vi "MAIN - PECT - Autonics - Pulses - encoder - Yokohama.vi"() -> ()   [LabVIEW 2018]
uses:
  Control 1.ctl
  <vilib>/DAQmx/read.llb/DAQmx Read (Counter U32 1Chan 1Samp).vi
  <vilib>/DAQmx/write.llb/DAQmx Write (Analog 1D Wfm NChan NSamp).vi
  <vilib>/DAQmx/read.llb/DAQmx Read (Analog 1D Wfm NChan NSamp).vi
  <vilib>/DAQmx/create/channels.llb/DAQmx Create Channel (AI-Voltage-Basic).vi
  <vilib>/DAQmx/create/channels.llb/DAQmx Create Channel (CI-Count Edges).vi
  <vilib>/DAQmx/miscellaneous.llb/DAQmx Fill In Error Info.vi
  <vilib>/DAQmx/configure/timing.llb/DAQmx Timing (Sample Clock).vi
  <vilib>/DAQmx/configure/trigger.llb/DAQmx Start Trigger (Digital Edge).vi
  <vilib>/DAQmx/create/channels.llb/DAQmx Create Channel (AO-Voltage-Basic).vi
  Global_data.vi
  <vilib>/measure/maspectr.llb/FFT Power Spectrum and PSD for 1 Chan.vi
  <resource>/objmgr/daqmx.rc
  <vilib>/Platform/NI_3dgraph.lvlib
  <vilib>/Instr/_visa.llb/VISA Configure Serial Port (Instr).vi
  <vilib>/measure/NI_MAPro.lvlib
panel:
  out "Array":dbl[][](array[numeric])
  in  "Filter 2":bool
  in  "low cutoff freq: fl 2":dbl=40.0 format="%0.2f"
  in  "Backdata":bool
  out "Numeric 2":i32
  out "Init pulses":i32
  in  "Motor counter":tag="Dev1/ctr0"
  in  "Motor Counter Terminal":tag="PFI8"
  out "dy":dbl[][](array[numeric])
  in  "2D Array In":dbl[][](array[numeric])
  out "Output":dbl[][](array[numeric])
  out "Current  Position (mm)":dbl=12.5
  out "Acquire":bool=TRUE
  out "Numeric":dbl=22.0
  out "Enum":T1(ring)
  in  "Direction (+)":string="+"
  in  "Tab Control 3":enum32{"Control", "Data Processing"}(tab)
  in  "Encoder":bool
  in  "Home":bool
  in  "Exit":bool
  in  "Scan":bool
  in  "Move Dis(mm)":dbl=150.0
  in  "Right":bool
  in  "Forward":bool
  in  "Left":bool
  in  "Backward":bool
  in  "Stop":bool
  in  "Pulser Trigger":tag="/Dev1/PFI0"
  in  "Edge":i32(ring)=10280 items=["Rising"=10280, "Falling"=10171]
  in  "2 Plots":bool
  in  "Offset":bool
  in  "Open csv":bool
  in  "Save Scan mode":bool caption="Save Process"
  in  "Gate 1":dbl
  in  "Gate 2":dbl=20.0
  in  "Open tdms":bool
  in  "Tab Control 4":enum32{"Basic", "Gaussian", "Chirp"}(tab)
  in  "Pulse Basic":T3={"Basic amp"=1.0, "Duty cycle %"=50.0, "Basic freq (Hz)"=200, "Basic Type"=2} {"Basic Type" items=["Sine Wave", "Triangle Wave", "Square Wave", "Sawtooth Wave"]; "Duty cycle %" format="%#.2f"; "Basic amp" format="%0.2p"}
  in  "Pulse Gaussian":T4={"Gauss amp"=2.8, "Gauss Nor. Band"=0.5, "Gauss atten (dB)"=6.0, "Gauss freq (Hz)"=1000.0}
  in  "Pulse chirp":T5={"Chirp amp"=2.1, "Chirp f2"=1500.0, "Chirp f1"=500.0} {"Chirp f1" format="%0.2f"; "Chirp f2" format="%0.2f"; "Chirp amp" format="%0.2f"}
  out "Motor Pulses":i32
  in  "Start idx":i32
  in  "End idx":i32=2000
  in  "Cursor":bool=TRUE
  in  "Repair Line Col":bool
  in  "Repair Line Row":bool
  in  "Line Col":dbl=167.0
  in  "Line Row":dbl
  in  "Y-max":dbl=55.0
  in  "Y-min":dbl
  in  "X-max":dbl=319.0
  in  "X-min":dbl
  in  "Inverse":bool caption="Scan"
  in  "ViewMode":i32(ring) items=["cwViewXYPlane", "cwViewXZPlane", "cwViewYZPlane", "cwViewUserDefined"]
  in  "Plot style":i32(ring)=5 items=["cwLine"=1, "cwPoint"=2, "cwLinePoint"=3, "cwHiddenLine"=4, "cwSurface"=5, "cwSurfaceLine"=6, "cwSurfaceNormal"=7, "cwContourLine"=8, "cwSurfaceContour"=9]
  in  "ColorMapAutoScale":bool=TRUE
  in  "Max":dbl=0.6
  in  "Min":dbl=-0.8
  in  "low cutoff freq: fl":dbl=40.0 format="%0.2f"
  in  "Filter":bool caption="Scan"
  in  "Backindex":i32
  in  "Backdata":bool caption="Scan"
  in  "Odd":bool caption="Scan"
  in  "DiffX":bool caption="Scan"
  in  "DiffY":bool caption="Scan"
  in  "Abs":bool caption="Scan"
  in  "Trim data":bool caption="Scan"
  in  "Return":bool caption="Scan"
  out "No.data":i32
  in  "Tab Control 2":T6(tab)
  out "Hall sensors signal 2":waveform(dbl)(graph)={"t0"=timestamp(3839287492.784824 s since 1904-01-01), "dt"=0.002, "Y"=[], "attributes"=variant("NI_ChannelName"=variant(string "Acquisition Task2"), "NI_UnitDescription"=variant(string "Volts"))}
  out "Hall sensors signal":waveform(dbl)[](graph)=[{"t0"=timestamp(3839287492.7848015 s since 1904-01-01), "dt"=0.002, "Y"=[], "attributes"=variant("NI_ChannelName"=variant(string "Acquisition Task0"), "NI_UnitDescription"=variant(string "Volts"))}, {"t0"=timestamp(3839287492.7848015 s since 1904-01-01), "dt"=0.002, "Y"=[], "attributes"=variant("NI_ChannelName"=variant(string "Acquisition Task0"), "NI_UnitDescription"=variant(string "Volts"))}]
  out "Feature Extraction":dbl(graph)=nan
  out "Power spectral density":cluster{"f0":dbl, "df":dbl, "magnitude":dbl[]}[](graph)=[{"f0"=0.0, "df"=inf, "magnitude"=[]}, {"f0"=0.0, "df"=inf, "magnitude"=[]}]
  in  "Add LF":bool
  in  "Save LF":bool caption="Save Process"
  out "Save Status":bool
  in  "3D Surface (":refnum<k7>(container)
  out "Record path":path=path "H:/Pulsed Eddy Current/PECT_default.tdms" caption="selected path"
  out "Feature extraction scan":dbl[](graph)
  in  "View Mode":bool caption="Scan"
  out "Hall sensors signal lf":dbl[][](graph)=[[-0.70660846198, -0.716567731313, -0.71772803455, -0.717921418426, -0.720596562008, -0.722079171705, -0.724657623384, -0.723561781416, -0.729298836376, -0.728847607304, -0.733553281611, -0.731232675116, -0.734068971955, -0.734230125187, -0.734649123582, -0.735197044564, -0.737292036575, -0.735906118769, -0.738162264033, -0.736454039766, -0.735454889741, -0.737968880154, -0.735422659102, -0.737292036581, -0.734552431644, -0.735809426849, -0.731909518652, -0.731264905752, -0.726591462081, -0.727171613726, -0.72340062815, -0.721080021693, -0.715278505501, -0.71253890069, -0.707188613582, -0.701870557272, -0.697068191179, -0.692362517146, -0.687946918849, -0.677826496722, -0.674571201711, -0.663773936246, -0.660776486438, -0.651622983945, -0.644113244288, -0.636120045089, -0.629867300614, -0.618425422989, -0.610399993434, -0.59950603696, -0.59218968167, -0.58322956384, -0.571207535404, -0.564471331877, -0.553126147145, -0.546615558225, -0.534915836753, -0.528792015616, -0.520315358066, -0.514803919133, -0.504103347861, -0.497753912499, -0.490534250062, -0.48415258421, -0.4781254554, -0.472839631231, -0.469197569495, -0.467811652195, -0.46571666097, -0.462429136198, -0.467457115235, -0.467231500771, -0.474354471106, -0.474741238726, -0.482927820085, -0.490469788806, -0.499204291135, -0.509066865834, -0.523216115386, -0.534432377128, -0.554350911396, -0.569177005115, -0.58816085171, -0.612366062487, -0.634250667901, -0.66187232831, -0.688269225307, -0.719081721676, -0.746928999864, -0.781093486223, -0.813130751347, -0.851227380515, -0.888357092222, -0.928000797226, -0.965807357181, -1.008351826422, -1.048994689492, -1.09189370194, -1.13485717869, -1.180109036257, -1.2251352826, -1.266293851833, -1.314639865003, -1.35380013893, -1.401147008934, -1.441370901989, -1.48307740981, -1.522592234217, -1.561881446939, -1.594208832793, -1.628276678402, -1.656575231322, -1.685228323683, -1.708627813295, -1.726709237842, -1.745338585167, -1.754749951221, -1.765386084343, -1.766481928394, -1.766578620469, -1.759068865834, -1.749141808352, -1.726870391409, -1.702697363978, -1.672142659225, -1.635496354594, -1.591855992024, -1.542736415895, -1.486816169566, -1.426544787201, -1.357119898907, -1.281152192711, -1.205055574576, -1.115615471107, -1.027496838527, -0.924487655795, -0.823476790057, -0.71266782326, -0.598377964549, -0.477738687781, -0.356454816131, -0.226146385508, -0.096933813379, 0.039691785785, 0.177477671952, 0.315553620416, 0.456562543074, 0.59605661768, 0.738386978448, 0.878138885599, 1.019921318004, 1.154935322631, 1.292076548544, 1.418613908244, 1.546504957955, 1.665822671713, 1.781143796386, 1.887472587349, 1.990352709737, 2.080759590593, 2.164752584475, 2.235692182322, 2.298122899903, 2.352689348501, 2.387788500997, 2.419503438832, 2.429204857999, 2.432524612792, 2.418181983039, 2.390753718718, 2.346694452024, 2.29477091497, 2.222380935278, 2.137904477937, 2.035346650361, 1.920347813654, 1.791425361517, 1.644195932762, 1.485299034053, 1.310738069287, 1.125154243505, 0.921650202866, 0.71092650171, 0.483765177519, 0.253445229601, 0.008105779367, -0.246129373952, -0.508261099919, -0.779449723152, -1.058244889529, -1.341584711586, -1.635528585329, -1.928441259944, -2.223868134907, -2.526772774422, -2.823650514512, -3.124106146674, -3.41405481644, -3.706227714753, -3.987442417835, -4.263822791101, -4.527407776882, -4.786577416573, -5.02840704592, -5.262275871216, -5.475098028081, -5.677574208879, -5.860454027961, -6.026509320014, -6.174450790588, -6.300217254762, -6.406645020668, -6.487352250666, -6.552781862445, -6.587011551361, -6.605834660103, -6.593973522799, -6.560743004097, -6.502017506172, -6.420568948967, -6.309918874295, -6.178350774499, -6.019772990024, -5.841921080871, -5.636479455639, -5.407702708707, -5.163100759281, -4.889329996495, -4.60340849308, -4.29102572782, -3.966589007543, -3.624329025262, -3.267791211866, -2.894429352616, -2.512784620922, -2.118957082525, -1.720230866355, -1.310095339563, -0.893610688781, -0.473226398891, -0.047749885035, 0.377081857903, 0.806651402224, 1.226326113266, 1.646645459066, 2.057327931374, 2.465367624173, 2.856937640696, 3.240772514315, 3.608041067282, 3.955230157274, 4.293975068757, 4.609804197942, 4.90271751193, 5.177098363499, 5.426887322034, 5.649860408204, 5.851142279943, 6.021772700426, 6.172194436626, 6.288354759714, 6.38169561436, 6.443353457295, 6.479452149573, 6.483029788153, 6.46127387881, 6.407834927929, 6.330674003129, 6.221217696105, 6.086943623705, 5.925176659162, 5.736206928573, 5.524965806055, 5.286167477957, 5.029771319924, 4.744593282131, 4.446168641795, 4.123506733751, 3.788113950506, 3.432351621052, 3.06650133258, 2.685180548865, 2.296898136162, 1.899107838935, 1.494871524426, 1.086445286821, 0.675762909712, 0.265467248353, -0.150952337452, -0.55870204758, -0.972221258056, -1.373654237756, -1.777923829368, -2.168979184481, -2.552460698049, -2.920729689806, -3.280071163481, -3.622008401497, -3.950860315772, -4.258117910152, -4.550936409787, -4.823256343074, -5.072595856712, -5.304498634402, -5.509682053404, -5.698202166799, -5.859132548236, -6.000240858013, -6.111889905191, -6.206424214181, -6.27008099717, -6.315365963394, -6.333898960157, -6.329676659853, -6.305148642671, -6.25857442753, -6.185216035338, -6.09506518857, -5.986381425725, -5.856360663809, -5.709708700472, -5.54117189352, -5.365641079165, -5.166356100054, -4.957401996174, -4.734878834588, -4.502332058483, -4.25769890765, -4.007715673153, -3.745098175872, -3.482835479658, -3.212193012196, -2.937618633024, -2.664784953904, -2.386601188071, -2.116185239442, -1.843835631437, -1.575257184583, -1.307226809354, -1.048865766862, -0.789924683906, -0.543553647601, -0.298858680926, -0.065186650983, 0.160975596988, 0.377855392589, 0.583937909112, 0.777321550784, 0.961906228802, 1.129988834268, 1.286113886493, 1.434406905534, 1.559977352138, 1.681841284773, 1.782239637185, 1.87196966226, 1.947711605492, 2.009916693762, 2.057166778279, 2.095037754511, 2.114505048262, 2.126913836672, 2.123561852274, 2.106834160961, 2.083724807448, 2.04517698859, 1.999828510872, 1.941362174369, 1.876127411384, 1.800417702224, 1.720518017024, 1.626759173182, 1.53477301667, 1.432666452766, 1.3256930704, 1.216753623473, 1.100658983649, 0.982533816097, 0.864892106737, 0.741448886061, 0.618489120633, 0.497011957912, 0.371215886709, 0.252865078568, 0.127455756566, 0.00929831228, -0.108053378055, -0.221569636608, -0.333216531681, -0.440351151746, -0.547066787125, -0.643984321714, -0.742481170629, -0.834016212751, -0.919943133402, -1.004129610016, -1.078743591058, -1.154131117554, -1.220526296559, -1.28176457554, -1.335299729295, -1.389318348703, -1.430928160202, -1.472151206875, -1.504381894686, -1.533711822363, -1.557723687612, -1.576417489536, -1.58798830868, -1.597464132915, -1.601750815379, -1.601621892616, -1.59852774587, -1.588246154234, -1.580027327232, -1.560882295453, -1.54560494743, -1.52268892626, -1.50177120885, -1.474117278751, -1.447236886611, -1.415296278632, -1.385869665753, -1.349996918726, -1.315800169399, -1.280926577982, -1.245472836775, -1.210728172549, -1.170472066246, -1.137048863988, -1.097276222791, -1.065400096546, -1.027077839927, -0.994814949512, -0.958942227201, -0.927646259992, -0.892128078709, -0.861283343899, -0.830664225057, -0.801817793355, -0.772777978979, -0.746928999873, -0.722723784605, -0.697132652466, -0.677504190288, -0.654072512801, -0.640019952773, -0.620713798494, -0.607112468066, -0.589804614323, -0.577589201926, -0.565986171871, -0.555930212629, -0.54590648416, -0.539105819592, -0.533239843546, -0.528050710938, -0.523635113662, -0.51996082103, -0.521346738438, -0.518703826188, -0.521314507795, -0.519896359761, -0.525472259972, -0.524408648935, -0.530177933006, -0.532079540602, -0.538815743842, -0.541813193149, -0.548871702871, -0.55319060837, -0.559572274784, -0.565953941223, -0.570885229012, -0.57865281302, -0.584647711969, -0.594349134521, -0.597120969574, -0.607305851908, -0.611399143265, -0.6213584113, -0.626902081599, -0.634282898507, -0.640019952747, -0.647046232714, -0.651300677507, -0.657295577056, -0.662162404096, -0.668737455294, -0.674216664635, -0.675602582331, -0.683531320648, -0.684949468998, -0.693136052559, -0.694167433224, -0.700516870141, -0.703095321724, -0.708961299059, -0.708219994242, -0.711443058732], [-0.711700903907, -0.720274255531, -0.721080021681, -0.724464239466, -0.722433708801, -0.725141083016, -0.72559231207, -0.726204694336, -0.729202144406, -0.727848457275, -0.731039291205, -0.729975679907, -0.73139382833, -0.73123267509, -0.734165663872, -0.732392978358, -0.735648273607, -0.732908668699, -0.73590611877, -0.734810276807, -0.73352105101, -0.733843357422, -0.732844207425, -0.733230975136, -0.731007060611, -0.73062029283, -0.728106302452, -0.729427758908, -0.724174163692, -0.726043541112, -0.72166017329, -0.721208944256, -0.715181813577, -0.712248824884, -0.70754315068, -0.704739084581, -0.697809495981, -0.693361667074, -0.688849376879, -0.681694173927, -0.676311656471, -0.666481310252, -0.663677244331, -0.654942740122, -0.649270147063, -0.638827419012, -0.632703597094, -0.62161625644, -0.613816441327, -0.601891104324, -0.593382215333, -0.583906407255, -0.574301676729, -0.564729176965, -0.553480684115, -0.54616432927, -0.535624910724, -0.527373867557, -0.517382370077, -0.511258549117, -0.498881984754, -0.493789544277, -0.484603813104, -0.479898140329, -0.472710708686, -0.46910087758, -0.464072898546, -0.462042368558, -0.459721762867, -0.45836807625, -0.458948227649, -0.460366375577, -0.465104278851, -0.467167039506, -0.476352770465, -0.481703055936, -0.495368845435, -0.504619038035, -0.520702125685, -0.534819144789, -0.554447603261, -0.570530691961, -0.592511988075, -0.615621357208, -0.640535643041, -0.667319306976, -0.694973199311, -0.727912918571, -0.7584675715, -0.795017126404, -0.828988231267, -0.870404618505, -0.908050021807, -0.951432484146, -0.989754736086, -1.033685125354, -1.077228749861, -1.121674836208, -1.166572155322, -1.211276093955, -1.257140340429, -1.302521130597, -1.347934155322, -1.389930731637, -1.437535450536, -1.478565113577, -1.521947620419, -1.557949302468, -1.598431053803, -1.629565906268, -1.663762677273, -1.691223234113, -1.718941638241, -1.740310595099, -1.759874633465, -1.772831377568, -1.782081590668, -1.788237655914, -1.788173194541, -1.784176586682, -1.7728636083, -1.758134175287, -1.733090917251, -1.706693971085, -1.669886510205, -1.632917898781, -1.584314009521, -1.53206805716, -1.471442131748, -1.407141915873, -1.333398119264, -1.254561886613, -1.168796071461, -1.07871136044, -0.983147451101, -0.877076363675, -0.77200444347, -0.655490661079, -0.541426425506, -0.414760028952, -0.290317564379, -0.158687687189, -0.026832212351, 0.113370977212, 0.253509690839, 0.395968995891, 0.538202675996, 0.682209031094, 0.82640876359, 0.965999515658, 1.107943100394, 1.2432149505, 1.379195876537, 1.506635696159, 1.632560682823, 1.748236342269, 1.865201233481, 1.969338348306, 2.067416114716, 2.15692054372, 2.236530178481, 2.30560040478, 2.364485757723, 2.409930942223, 2.44470779056, 2.468332842109, 2.474327739345, 2.470137757407, 2.448124237269, 2.417408447956, 2.366355134083, 2.304955792292, 2.22576515062, 2.134197956683, 2.022454403625, 1.899978065497, 1.759420364327, 1.606872887466, 1.438564653815, 1.256074962083, 1.059951729476, 0.851161868759, 0.630478906609, 0.399030903911, 0.159009529445, -0.095741280337, -0.355101129604, -0.628997073303, -0.906148413194, -1.193065765257, -1.484979020361, -1.782984050494, -2.083052046727, -2.385956572993, -2.689473733606, -2.994473784422, -3.295767585382, -3.589680826897, -3.885270392832, -4.167097682705, -4.447442674322, -4.711382413403, -4.969939881134, -5.21305896681, -5.445155293591, -5.65475453306, -5.853298698642, -6.032053093797, -6.193563935177, -6.333222102904, -6.451672172544, -6.551138064005, -6.625721405834, -6.678709764359, -6.705397338156, -6.7118436127, -6.689732892102, -6.647219721964, -6.571991743565, -6.476812606234, -6.354849306761, -6.207552308847, -6.03563076211, -5.840825219647, -5.620911798473, -5.380693017663, -5.114625193963, -4.828993469243, -4.526666463854, -4.200843492433, -3.861516208625, -3.502302924475, -3.13216385381, -2.744427224852, -2.350406050506, -1.943944235937, -1.534034129331, -1.111328792601, -0.688108072092, -0.254348183817, 0.180185043615, 0.614653678333, 1.048574325895, 1.479626447166, 1.903394510606, 2.321264488474, 2.731753822843, 3.124806592014, 3.511768013492, 3.874782309212, 4.221391454251, 4.556655670645, 4.868101642753, 5.155503714809, 5.423470852265, 5.66481553335, 5.882245096744, 6.070795930585, 6.233626609533, 6.371091627426, 6.475326584487, 6.555807348401, 6.601285277357, 6.622976737884, 6.609955415071, 6.570891451368, 6.499628742443, 6.407544849292, 6.28052263845, 6.128070288235, 5.948608528303, 5.743491108137, 5.514426315553, 5.258964657354, 4.982101962969, 4.683548195569, 4.366655388863, 4.026975726542, 3.675113132109, 3.302687625615, 2.924912076204, 2.52876527563, 2.127365065353, 1.717166033533, 1.303228338131, 0.883199090654, 0.465587113791, 0.041722314718, -0.374858506392, -0.792632058415, -1.209664560433, -1.619703313065, -2.022973968836, -2.416640254231, -2.801153418931, -3.170164003204, -3.529376856542, -3.867414465728, -4.195654308351, -4.499141189584, -4.786964188961, -5.051871271029, -5.297149939141, -5.518352233991, -5.717154105289, -5.893104251006, -6.046299304766, -6.173645008773, -6.275238003521, -6.35791128069, -6.408675593623, -6.444194505839, -6.448062264612, -6.433687095446, -6.394268196495, -6.335252674733, -6.248389341404, -6.145345955566, -6.020353152397, -5.879180364564, -5.71757311064, -5.538109933487, -5.346721406584, -5.136058870085, -4.916694164197, -4.681472020658, -4.438804768894, -4.185340402521, -3.926783816261, -3.653465746224, -3.381437188134, -3.103252801735, -2.823908360859, -2.542275774546, -2.258999645662, -1.980912873448, -1.705791511432, -1.431605004604, -1.161544171119, -0.901281584442, -0.641986021923, -0.394615883648, -0.147374738228, 0.083364272888, 0.312008253063, 0.526470734451, 0.730973938979, 0.921811355892, 1.10391427476, 1.267806902505, 1.422997270747, 1.563135951752, 1.687868408833, 1.801094545084, 1.89701284902, 1.981811596561, 2.050430579225, 2.106834160953, 2.147799278231, 2.17816052264, 2.190633772981, 2.194823753727, 2.183317421989, 2.162238596067, 2.128299753321, 2.084208266714, 2.0311889008, 1.967017743996, 1.893370789696, 1.81256864297, 1.725739375948, 1.627307093536, 1.528359125728, 1.41655114942, 1.30799846779, 1.188100615371, 1.068557301022, 0.944695085629, 0.822992319382, 0.695069043221, 0.570272131299, 0.442284382926, 0.317616379586, 0.194624359058, 0.068441497018, -0.050553949051, -0.171128708146, -0.285160663856, -0.399676092901, -0.508132177389, -0.615073436322, -0.712184363585, -0.810874605876, -0.899960127607, -0.986692823527, -1.067462858994, -1.142721461342, -1.214112393046, -1.278251431973, -1.337298031367, -1.389382810045, -1.440339520092, -1.481240260618, -1.520884007654, -1.548602401773, -1.57802902429, -1.595723675412, -1.612902636098, -1.621959461795, -1.628502293261, -1.629275830005, -1.627986602099, -1.618188470277, -1.608358107981, -1.59524021497, -1.575482799408, -1.556627844048, -1.531455674043, -1.507895039751, -1.477243655394, -1.44794596169, -1.414168204733, -1.38277552038, -1.345710238439, -1.31270602436, -1.274061444278, -1.238059782054, -1.200704434038, -1.16164086315, -1.124865672142, -1.086188874377, -1.050283915983, -1.013218656049, -0.978731850936, -0.941376519413, -0.91175654708, -0.874530142074, -0.846586166678, -0.814258824097, -0.786379312543, -0.757500652045, -0.731554981564, -0.705641542641, -0.684433778674, -0.659003801079, -0.639955491476, -0.622712098238, -0.603212560587, -0.590352535192, -0.573463680108, -0.562601954829, -0.551933613494, -0.542554497827, -0.532853075905, -0.529694473448, -0.52025089677, -0.519058363199, -0.513837000046, -0.511451932947, -0.512870080968, -0.511838700566, -0.511677547393, -0.514352690234, -0.517285678205, -0.520508741861, -0.526568101624, -0.527825096497, -0.538493437484, -0.540427275726, -0.547389093516, -0.553061685838, -0.559540044149, -0.566147325069, -0.57620328444, -0.578652813016, -0.588676541915, -0.596540818049, -0.602116718805, -0.61207598672, -0.616749429656, -0.626450852631, -0.6339605921, -0.639955491487, -0.645563623199, -0.654459280486, -0.657263346399, -0.666739155394, -0.66922091493, -0.67573150487, -0.681823096537, -0.68501393027, -0.690783215552, -0.69532773638, -0.698035110534, -0.70357878138, -0.706382847481, -0.706995229747, -0.714827276494, -0.711829826488, -0.717115652296], [-0.710927368415, -0.721563481368, -0.721595712031, -0.723303936229, -0.725108852432, -0.725527850816, -0.729427758978, -0.727300536363, -0.732876438089, -0.733166513892, -0.737034191399, -0.735003660722, -0.738549031766, -0.738452339841, -0.737968880135, -0.738903568875, -0.741095252863, -0.738645723707, -0.741030791566, -0.739677104411, -0.739354797941, -0.742094402897, -0.73774326562, -0.742932399702, -0.737743265618, -0.738968030203, -0.735519351038, -0.735035891386, -0.730845907349, -0.72978229604, -0.724464239482, -0.723819626589, -0.716019810351, -0.714408278121, -0.708574531326, -0.703063091172, -0.698679723421, -0.692878207473, -0.688398147883, -0.678213264461, -0.674829046864, -0.664257395879, -0.659519491377, -0.650656064667, -0.642179405778, -0.633799438886, -0.625226088263, -0.614525515429, -0.606081087604, -0.593478907265, -0.587516238926, -0.577041281088, -0.564471331913, -0.558605355655, -0.545197410173, -0.540781812775, -0.528276325465, -0.521250046516, -0.512773389061, -0.505295881372, -0.496013458178, -0.490598711337, -0.480768367493, -0.477255228246, -0.470325641713, -0.466393504254, -0.46226798305, -0.458819305132, -0.460559759439, -0.456659852641, -0.462429136215, -0.463879514767, -0.471389252665, -0.472517324904, -0.483153434512, -0.490502019438, -0.50084805357, -0.513160156676, -0.528147402851, -0.542361113995, -0.561699496934, -0.579780885408, -0.602664639692, -0.627611155718, -0.650108143758, -0.682467709413, -0.707704303918, -0.742610093227, -0.773390361308, -0.810391146154, -0.844877942157, -0.884070415338, -0.922714969748, -0.965130513384, -1.004194071312, -1.050251685316, -1.092699468449, -1.135695176079, -1.183235411066, -1.227133584269, -1.276382052832, -1.317637317973, -1.366466795995, -1.408012144306, -1.454714405619, -1.494777149486, -1.537934042904, -1.57635302815, -1.614095171865, -1.647905173327, -1.679620181747, -1.706984047416, -1.734025607719, -1.755845795159, -1.771058688734, -1.787077350425, -1.793910260671, -1.803063782041, -1.796939947333, -1.794844951197, -1.782500589886, -1.765353853546, -1.740826286392, -1.711657499304, -1.673367425821, -1.633207975063, -1.581703323307, -1.527845836705, -1.464705918282, -1.396151253222, -1.324856989698, -1.238930010223, -1.155291421567, -1.061242341096, -0.964228054985, -0.855095058719, -0.747960380555, -0.628481383047, -0.509260249656, -0.382271551645, -0.252317654314, -0.117787026094, 0.01909642047, 0.16013760098, 0.300663077532, 0.445829750017, 0.592833556893, 0.73248877748, 0.882199941889, 1.021210542207, 1.165829267176, 1.303453952372, 1.438274578348, 1.570484530423, 1.696796287823, 1.813857867449, 1.930307073514, 2.031124439534, 2.130330282341, 2.219673563048, 2.293578381865, 2.362261844503, 2.416119222821, 2.462434636828, 2.491828971774, 2.511876424447, 2.513326802871, 2.507525289189, 2.480902787945, 2.44390202482, 2.389980183652, 2.321103335349, 2.237626019648, 2.138613551575, 2.020552797226, 1.892371640636, 1.746141352558, 1.583860232908, 1.41087856266, 1.216528009233, 1.019792395584, 0.801139968617, 0.572592735082, 0.334891987588, 0.086426181539, -0.174448462454, -0.439416463364, -0.719307336175, -1.001099928024, -1.292304006338, -1.591630377162, -1.893019701465, -2.201209923647, -2.506660775153, -2.815625046101, -3.122430143612, -3.429364475269, -3.72505055753, -4.023057597177, -4.307076750992, -4.584972354295, -4.851974206402, -5.106148417387, -5.347559415797, -5.576948483823, -5.784839614889, -5.981159965478, -6.156111198496, -6.30959656147, -6.45041515099, -6.55987275788, -6.655793263995, -6.722995668099, -6.76869976497, -6.787490663209, -6.783590665282, -6.752519610718, -6.698564287283, -6.615794148269, -6.511880294189, -6.378281466584, -6.220025813415, -6.041238998862, -5.833121960323, -5.605054062077, -5.350234599383, -5.079590001991, -4.780034515432, -4.468360588381, -4.130322168267, -3.780036472621, -3.411089577322, -3.030185528628, -2.634907020607, -2.231700205315, -1.816117219547, -1.398761938448, -0.967870119262, -0.533948917579, -0.10031802868, 0.342014952778, 0.778997542299, 1.221878289721, 1.653542809478, 2.083595884971, 2.502368388148, 2.912342123176, 3.308199069955, 3.69280778213, 4.05759490835, 4.402173670004, 4.736986818805, 5.045499953056, 5.330420413114, 5.590007684748, 5.831030201483, 6.037340233968, 6.223796171648, 6.375088266782, 6.505817090897, 6.600028268508, 6.67061415748, 6.707615353626, 6.71873505223, 6.697236968676, 6.649148309384, 6.567990662195, 6.460919338063, 6.323744347412, 6.159398755148, 5.970042083259, 5.748390202495, 5.509785072288, 5.239207160015, 4.951933935452, 4.638650733591, 4.311863128522, 3.962482067337, 3.598823090781, 3.219435814265, 2.828187905105, 2.423532267353, 2.013268677874, 1.593787260336, 1.170857241583, 0.745058713974, 0.317455226524, -0.10628069381, -0.536559599228, -0.956170390698, -1.37877891595, -1.790010344895, -2.197890157421, -2.592974779821, -2.979196378686, -3.349786489195, -3.70845164637, -4.045715944667, -4.3717965508, -4.673607650656, -4.956273909006, -5.2199564235, -5.459272535097, -5.679089074392, -5.868286213282, -6.041658005013, -6.18408794079, -6.30775937747, -6.402938419599, -6.474846495158, -6.520550523301, -6.54420832557, -6.539824863307, -6.514362106984, -6.463887844289, -6.3946872037, -6.301667662811, -6.18431355981, -6.054260422905, -5.897584390787, -5.732012684015, -5.54088181332, -5.340758648073, -5.123682130552, -4.894293578911, -4.649466615545, -4.398161494277, -4.134189881976, -3.865738458211, -3.588165975379, -3.308531000887, -3.0243839815, -2.736756297111, -2.452932090653, -2.16456357347, -1.884962022521, -1.602911120461, -1.331432047928, -1.056794509731, -0.793631208497, -0.533046459727, -0.280068224611, -0.036372475961, 0.196300351006, 0.424912084094, 0.636344877161, 0.841073689194, 1.031073107354, 1.206472060374, 1.373845595888, 1.519656861632, 1.659795547723, 1.778468655645, 1.889341962949, 1.981070292399, 2.061356758571, 2.12433538713, 2.176226685399, 2.211293601344, 2.236240102863, 2.244781217885, 2.243040764236, 2.228472522925, 2.201495492363, 2.160498142613, 2.110605143374, 2.055104018764, 1.981038061762, 1.907165492431, 1.816758622552, 1.72515922494, 1.623342728618, 1.517207335446, 1.405012592267, 1.290142712201, 1.168246562564, 1.047156179274, 0.919039523837, 0.792727780462, 0.665803652141, 0.534979615125, 0.407733168748, 0.276586809842, 0.152950173688, 0.024575625662, -0.097675117694, -0.219539107163, -0.33276530288, -0.44750635248, -0.555833520716, -0.659648413935, -0.759434490888, -0.85722228175, -0.945888811272, -1.032557052242, -1.113939476566, -1.187393167446, -1.260202254478, -1.321988459376, -1.383935824916, -1.431895080745, -1.481530336808, -1.52059393143, -1.554532849089, -1.584926392742, -1.610227488406, -1.62624614447, -1.64239372398, -1.647872942625, -1.65280423958, -1.652836470222, -1.645584563108, -1.639911960213, -1.625472607776, -1.610549795346, -1.5874726176, -1.567940817251, -1.540705882338, -1.514212254869, -1.483045179111, -1.452554949714, -1.416521044576, -1.38277552039, -1.345001163501, -1.307291270799, -1.268163230894, -1.23274172125, -1.193581455997, -1.150585744158, -1.117291465704, -1.074875911501, -1.041484945369, -1.003001536946, -0.967515582024, -0.932223013107, -0.898219672272, -0.863507258885, -0.833178215835, -0.799142649494, -0.772745748364, -0.743351398115, -0.716471039411, -0.693587281637, -0.668092842444, -0.650688295345, -0.627256618724, -0.612881752772, -0.595863974652, -0.583519639569, -0.56724316682, -0.556800439871, -0.545551947147, -0.535721602628, -0.528276325388, -0.523796266856, -0.516060913979, -0.514094845139, -0.511065165314, -0.508841251385, -0.512032084435, -0.509002404553, -0.516350989715, -0.514513843417, -0.520831048233, -0.522764886451, -0.526729254832, -0.53195061806, -0.538590129407, -0.541652039967, -0.550966694366, -0.553802990491, -0.563053183779, -0.569853848527, -0.575590902357, -0.584905557093, -0.590932686735, -0.601020877055, -0.60350263635, -0.614944513774, -0.618908882582, -0.629125995866, -0.634927511342, -0.643146325024, -0.647884229412, -0.655651814247, -0.659551722015, -0.665675544213, -0.668963069777, -0.677633112898, -0.681629712678, -0.682854477157, -0.691717904228, -0.692169133285, -0.701097021755, -0.701580481458, -0.70715638295, -0.710379447476, -0.713634742606, -0.714279355512, -0.718340416815], [-0.711765365224, -0.724560931444, -0.722369247503, -0.726784845983, -0.72494769918, -0.728621992799, -0.727880687945, -0.730072371842, -0.730169063782, -0.730845907354, -0.730104602467, -0.732618592899, -0.730749215401, -0.73229628649, -0.731135983188, -0.734230125256, -0.735744965582, -0.730781446088, -0.737066422059, -0.732747515477, -0.736228425243, -0.735197044577, -0.734326817112, -0.734584662293, -0.73342435903, -0.730555831519, -0.730684754112, -0.725270005612, -0.726108002436, -0.721885787838, -0.717824726532, -0.717147883005, -0.710476139452, -0.711249674934, -0.703578781432, -0.702676323345, -0.696004579975, -0.692813746133, -0.684240394829, -0.67934133696, -0.672121672803, -0.663354937875, -0.655812967451, -0.650043682499, -0.638440651315, -0.632123445558, -0.622744328924, -0.611689219083, -0.607595927736, -0.593865674939, -0.589933536879, -0.575333057211, -0.567501011901, -0.558411971797, -0.547131248426, -0.538364514917, -0.530081241095, -0.517382370075, -0.51100070404, -0.498624139668, -0.492371396341, -0.485183964551, -0.476449462421, -0.473194168256, -0.465555507761, -0.464234051759, -0.457014389609, -0.457755694206, -0.454371477587, -0.456530930071, -0.456982158954, -0.458819305118, -0.462396905535, -0.46897195505, -0.47374208902, -0.483926969825, -0.492210243146, -0.508003254901, -0.522893809026, -0.535270373741, -0.558895431386, -0.574559521866, -0.601278722161, -0.624001323916, -0.650913909799, -0.679824796629, -0.710411678102, -0.740547331832, -0.775582045369, -0.808135000648, -0.848326621873, -0.884908412339, -0.925744651385, -0.968127964584, -1.008577441074, -1.056762279125, -1.097276222847, -1.147588292081, -1.191615385176, -1.241476233341, -1.284697567014, -1.33227004555, -1.378778915937, -1.420968878904, -1.465318301289, -1.510505725619, -1.547055328546, -1.589825458321, -1.625085839421, -1.659056995213, -1.6933182298, -1.717781332923, -1.748690578516, -1.765740622068, -1.785755891413, -1.798164714248, -1.806254622338, -1.809703308258, -1.809252078319, -1.799163866215, -1.788269886665, -1.76541831494, -1.743694819196, -1.711302961563, -1.672851734771, -1.630113828191, -1.577964562881, -1.525267381534, -1.456487093395, -1.391864572571, -1.311513489345, -1.230872342166, -1.140529775998, -1.045288163425, -0.943826049219, -0.836916971325, -0.721821326526, -0.606467855284, -0.479189066374, -0.355326744083, -0.223052245422, -0.083783719617, 0.049554354938, 0.196719348996, 0.334666373306, 0.48295941228, 0.627545921343, 0.774259643201, 0.919458521707, 1.065463162938, 1.206891058243, 1.34793218853, 1.481882589672, 1.615349537597, 1.739276232442, 1.860205488455, 1.972754793568, 2.073636624006, 2.174131695086, 2.255288400978, 2.334833581771, 2.396265156012, 2.453506752411, 2.495084265497, 2.524027372682, 2.541045146617, 2.543430213434, 2.529861117134, 2.506655062122, 2.462015638659, 2.408770639614, 2.335897192413, 2.24555475284, 2.146123286002, 2.021197409573, 1.891179107926, 1.737793624341, 1.575093507418, 1.394763259411, 1.202088698055, 0.994652523619, 0.776225710175, 0.544100877349, 0.304208444897, 0.047813901563, -0.211159144441, -0.483798047303, -0.7653326994, -1.052572293041, -1.351124992534, -1.647808481302, -1.959221597519, -2.263576411537, -2.577342854314, -2.887370806551, -3.196786672335, -3.502560771377, -3.804693114694, -4.097801143999, -4.386429416404, -4.661940020556, -4.932841925659, -5.185952608819, -5.425397603927, -5.655914855497, -5.862258976218, -6.060545516593, -6.229662966251, -6.387080614154, -6.520099284844, -6.631684206844, -6.718579969795, -6.784170830334, -6.823106351241, -6.840704694108, -6.828811308327, -6.796128675609, -6.733793179361, -6.64683294574, -6.537890983214, -6.395138442166, -6.238010868241, -6.046911698304, -5.838214491566, -5.598736752886, -5.34024295002, -5.058736491301, -4.756151316888, -4.432584187887, -4.093063195321, -3.731174427893, -3.358005356716, -2.96743213227, -2.568350468634, -2.160405808323, -1.73857013707, -1.318604238285, -0.881105195248, -0.447989812003, -0.002143557587, 0.439770395346, 0.884520545481, 1.326466604942, 1.764770645786, 2.195178290564, 2.620235815048, 3.02843692896, 3.430288857773, 3.814124125672, 4.179072505695, 4.52316791251, 4.853211018603, 5.164689498048, 5.44345397781, 5.704814050875, 5.9364897071, 6.144959296661, 6.322745187771, 6.475552201279, 6.596772938093, 6.691693235321, 6.755704025392, 6.790030060846, 6.791222608696, 6.766114644038, 6.710580606664, 6.62197757689, 6.508234414488, 6.359295095206, 6.193789165152, 5.98938063049, 5.765923803883, 5.515522164724, 5.241753395342, 4.94510100651, 4.628981503492, 4.290397456829, 3.93847018769, 3.564207334467, 3.179985482758, 2.78126008812, 2.368385663559, 1.953803191747, 1.525587293446, 1.098338380085, 0.665416884865, 0.236459696272, -0.197138822371, -0.624291399669, -1.052507831657, -1.472989204735, -1.890312321264, -2.296774081073, -2.696242198286, -3.081722610934, -3.457050786674, -3.813749999477, -4.153560682818, -4.479544743602, -4.778809735956, -5.065569480639, -5.322515831455, -5.562960158558, -5.776523965273, -5.966945991103, -6.133227000213, -6.275431391187, -6.390561595666, -6.484773744206, -6.547657079024, -6.589880141444, -6.607413996422, -6.599259464388, -6.570734721027, -6.512073682302, -6.438199480229, -6.338024566655, -6.220122507215, -6.078304936196, -5.921564420508, -5.743229139087, -5.550132156053, -5.341113190445, -5.117300374375, -4.880176376789, -4.633899033522, -4.373504792794, -4.106825808411, -3.833475315589, -3.551261620261, -3.269950678431, -2.976327836394, -2.691053042014, -2.398881106403, -2.110996091378, -1.823433590916, -1.540995958539, -1.262200556184, -0.990302657263, -0.720725484573, -0.461558909037, -0.206614626238, 0.037919101747, 0.272267907717, 0.499590406638, 0.709766199878, 0.914688392123, 1.100852367279, 1.279925610207, 1.440724104466, 1.590016279132, 1.724740227003, 1.845605020756, 1.949516519928, 2.042534077976, 2.117470265228, 2.181157970384, 2.227731218564, 2.261766756197, 2.283038967805, 2.28664879767, 2.282748892171, 2.259220536969, 2.232630273161, 2.185960332916, 2.134133495452, 2.069672257958, 1.998023596367, 1.916286756241, 1.827588108294, 1.729381434927, 1.628402934234, 1.516723876331, 1.403529984368, 1.285275890746, 1.159995527641, 1.038131609861, 0.904245675988, 0.777353781392, 0.643338918953, 0.515641249901, 0.383495749512, 0.254637762314, 0.12616653192, 0.001015043127, -0.123491846328, -0.242132776215, -0.360709259352, -0.471582636471, -0.580715573951, -0.687463459203, -0.785315701171, -0.884682797774, -0.971737798179, -1.062015877006, -1.138015783997, -1.214273546373, -1.282054651605, -1.345678007751, -1.402500697588, -1.453940869169, -1.497774603487, -1.539384423977, -1.570196965704, -1.599140129151, -1.621701616217, -1.638977270006, -1.65506038846, -1.657896689984, -1.66540644294, -1.659475994245, -1.6561884629, -1.644843256998, -1.631628670883, -1.614481940201, -1.594917908013, -1.569326736977, -1.543928951467, -1.513599871748, -1.483303024612, -1.44929965047, -1.4141037433800001, -1.380390449999, -1.340682252615, -1.307678038826, -1.264521164743, -1.230131036731, -1.189617083625, -1.151584894783, -1.112360173922, -1.07342553161, -1.034780967818, -0.998328091321, -0.959328995068, -0.926228111175, -0.88954962641, -0.857383435016, -0.825056091908, -0.790665988836, -0.767621075384, -0.735583812304, -0.713473589391, -0.685658543145, -0.665159853888, -0.642662865403, -0.622808790165, -0.604050557231, -0.587870775927, -0.571852148146, -0.55921773777, -0.545165179484, -0.536269523486, -0.526535870989, -0.517736907139, -0.515287378725, -0.507165258283, -0.507906562927, -0.501395974404, -0.503748810838, -0.50236289347, -0.504393423551, -0.505682649001, -0.508293330553, -0.510388321916, -0.515867530145, -0.518059213454, -0.524569802165, -0.52875978496, -0.535786063969, -0.544327182925, -0.5475180161, -0.558959892661, -0.561989572689, -0.574462829917, -0.58013542245, -0.588805464462, -0.597636659824, -0.605597627963, -0.612591676972, -0.619392342204, -0.625580625296, -0.63495974198, -0.639891030191, -0.646466081183, -0.654330357939, -0.658165804432, -0.668737455312, -0.669672143973, -0.680662793387, -0.683982549693, -0.691427828421, -0.694360817091, -0.698679723403, -0.703030860409, -0.706511770053, -0.708606761965, -0.712861207147, -0.712990129697, -0.717695803943, -0.718082571675], [-0.71427935551, -0.722143632976, -0.72404524108, -0.724464239483, -0.726011310473, -0.728170763755, -0.726236924985, -0.730974829944, -0.729911218611, -0.734423509066, -0.732006210595, -0.73532596716, -0.734326817122, -0.73645403979, -0.734487970348, -0.737324267224, -0.735809426843, -0.737130883336, -0.735616042946, -0.735841657505, -0.735809426825, -0.734004510669, -0.735325967138, -0.73245743967, -0.733005360631, -0.72833191696, -0.728944299233, -0.724367547531, -0.724883237855, -0.721015560384, -0.718179263577, -0.713151282924, -0.711636442602, -0.704996929745, -0.70048463953, -0.69590788798, -0.690009680114, -0.685787465724, -0.676247195206, -0.67276628568, -0.662742555697, -0.659003801098, -0.648496611662, -0.643371939515, -0.635346509704, -0.629125995852, -0.617587426319, -0.609626458033, -0.598313503252, -0.590062459426, -0.5810056497, -0.569982771092, -0.560764808435, -0.550934463727, -0.54278011233, -0.530435778128, -0.525568951902, -0.515126225547, -0.509163557759, -0.49820514143, -0.491275554701, -0.483862508508, -0.476868460633, -0.470647948067, -0.466232351115, -0.461107680184, -0.458625921328, -0.455628472316, -0.453501250461, -0.455789625498, -0.455499549774, -0.462267983033, -0.463879514753, -0.471679328402, -0.477351920158, -0.487569031621, -0.495787843706, -0.511451932955, -0.524118573203, -0.541361964245, -0.557606205819, -0.579490809668, -0.601020877026, -0.62522608831, -0.651203985583, -0.68021156439, -0.710701753907, -0.739967180224, -0.77648450352, -0.809585379893, -0.849261310757, -0.886810020881, -0.928903255565, -0.969288268192, -1.013669885247, -1.056182127116, -1.102239745154, -1.14662137207, -1.194193838741, -1.239993622437, -1.283891800131, -1.333108043207, -1.377167381948, -1.425126637116, -1.467606680147, -1.512761873853, -1.55398492737, -1.595369137754, -1.630146058852, -1.665793211348, -1.697089221818, -1.725935700923, -1.7511078814, -1.771961148467, -1.789784729985, -1.802322475745, -1.811443766655, -1.812088380825, -1.814022223456, -1.80486870181, -1.794780489812, -1.772154532753, -1.749109577661, -1.716040874956, -1.677847493227, -1.632305515562, -1.582380167971, -1.52243108076, -1.459226701699, -1.386159741905, -1.308967265931, -1.22658566283, -1.13463156401, -1.040292410915, -0.936348537068, -0.829181615174, -0.712764515191, -0.595606129522, -0.467747190914, -0.342724567549, -0.20651793436, -0.070891470967, 0.071600097559, 0.213414807264, 0.359129407496, 0.506584448778, 0.654297325408, 0.800882123762, 0.94737022586, 1.096952464068, 1.236027525487, 1.379518182597, 1.512469436124, 1.645259542865, 1.769379623202, 1.890341111973, 2.001085504894, 2.107930002, 2.202365719158, 2.290387550084, 2.363937837082, 2.429043704874, 2.484931616791, 2.523350529433, 2.553260556559, 2.564992507132, 2.567732111023, 2.551584563608, 2.522383610465, 2.476454960925, 2.420470357663, 2.343825926324, 2.255417323432, 2.149281886744, 2.02712784304, 1.88930973233, 1.737761393734, 1.570162224343, 1.387124605696, 1.192451747079, 0.979407447398, 0.758434415577, 0.519895690267, 0.278069418051, 0.018709653029, -0.244840148886, -0.519219516403, -0.800979796488, -1.094955614997, -1.389286118006, -1.694833072763, -2.000702537671, -2.312986148011, -2.625850171815, -2.93652278559, -3.249355170025, -3.556031789992, -3.859840201111, -4.153141680389, -4.444058420266, -4.719923636027, -4.989923143988, -5.243775212777, -5.485573151627, -5.709837625206, -5.920081784168, -6.110826273553, -6.282651200402, -6.433461476219, -6.566415720895, -6.675067619843, -6.758450185193, -6.824588995507, -6.859173286962, -6.875772460093, -6.859624526589, -6.824137755937, -6.759191506871, -6.670909773554, -6.553490951991, -6.413091283668, -6.242394322554, -6.052036466714, -5.835281451458, -5.593354147693, -5.330863692688, -5.043555652639, -4.739294486152, -4.410602654685, -4.067600751817, -3.704519477413, -3.328385203867, -2.933009627492, -2.530962774319, -2.115669547686, -1.693124845495, -1.263489783148, -0.828827078002, -0.386300380611, 0.058256621803, 0.505617530523, 0.952494892089, 1.394537645167, 1.835839145116, 2.264699742945, 2.692754748947, 3.102277361797, 3.50377480462, 3.887610130214, 4.256039492337, 4.596750738449, 4.933014458055, 5.236660924787, 5.523160877875, 5.777881462885, 6.010846419604, 6.2183169114, 6.393878919235, 6.543752959125, 6.662072941399, 6.755220560184, 6.813171935692, 6.845145114857, 6.842824480732, 6.813043011561, 6.751642917357, 6.662395251416, 6.541206711077, 6.393330992815, 6.217124366535, 6.015197593409, 5.783360713855, 5.527576505504, 5.25171272113, 4.94664808477, 4.627563349858, 4.28085715874, 3.924030829939, 3.544707770738, 3.153072880645, 2.747514606141, 2.33567157803, 1.91096870489, 1.484364346433, 1.050250317358, 0.616329669921, 0.182570109135, -0.253639110055, -0.683982549674, -1.11674354445, -1.538546426072, -1.960156288454, -2.37003457972, -2.77282255144, -3.157593978725, -3.533856947913, -3.889943875657, -4.232300908653, -4.554030586337, -4.856518784492, -5.137799349038, -5.398001136619, -5.634513353977, -5.846497912768, -6.037081168104, -6.199268870824, -6.342891493272, -6.452542418278, -6.544337250969, -6.604609868697, -6.644834601269, -6.655342024898, -6.646123855617, -6.609670191078, -6.552620705694, -6.468625849124, -6.367838522832, -6.242458785089, -6.09641890151, -5.935520541452, -5.752995191112, -5.558125484081, -5.340597492477, -5.116043361895, -4.87360124189, -4.623746263204, -4.360483476925, -4.091000415003, -3.811332681458, -3.529409087399, -3.23955699438, -2.947416799028, -2.655115719545, -2.362782659945, -2.072834905165, -1.782017129298, -1.498902677582, -1.216852000067, -0.94714580684, -0.674474509818, -0.416436021814, -0.161008292115, 0.081430435869, 0.318454375505, 0.544294261008, 0.759046797099, 0.958908782521, 1.150551960331, 1.3256930704, 1.486878333803, 1.635815974349, 1.76644663758, 1.890308881358, 1.990932860833, 2.080437284391, 2.153504097989, 2.215451351557, 2.258769308244, 2.293352767506, 2.308662314137, 2.315462975972, 2.305793788522, 2.284328192747, 2.252226491756, 2.205878856903, 2.151119032095, 2.086722254951, 2.012656296172, 1.924892330287, 1.837353983908, 1.733055724553, 1.631819378809, 1.517948639422, 1.40256306617, 1.282407366842, 1.158480689198, 1.028752503791, 0.90166722756, 0.766975526221, 0.637891946316, 0.507035677319, 0.372086113208, 0.24358266189, 0.112178444411, -0.013037507026, -0.137544398039, -0.257474554668, -0.376889036173, -0.487536800959, -0.600956415756, -0.703159783003, -0.806040008442, -0.902216273391, -0.990496041248, -1.076519675291, -1.157612029636, -1.230034344694, -1.299201370965, -1.362437961015, -1.417391273061, -1.472054514814, -1.511633799747, -1.553630389705, -1.586860234387, -1.614417478835, -1.637397965769, -1.654061236775, -1.663472600955, -1.673560810025, -1.673045118824, -1.670337740007, -1.664310599148, -1.651837318588, -1.640621035564, -1.618220700996, -1.597947593358, -1.574483647939, -1.548860247294, -1.515694866593, -1.488202089125, -1.451394645029, -1.4187771924249999, -1.379552452264, -1.342003710407, -1.304745047244, -1.26558477698, -1.224361746464, -1.185652711274, -1.144719762673, -1.105301658294, -1.069815697357, -1.028044759736, -0.99458933488, -0.955622469533, -0.920974514364, -0.885778639949, -0.851807532229, -0.818900037683, -0.789795761301, -0.758145264994, -0.731458289609, -0.704674623302, -0.678825646667, -0.658520341464, -0.634411821073, -0.617297350552, -0.598152350062, -0.584067560455, -0.566953091032, -0.556284749658, -0.54139419487, -0.533626611202, -0.523312807272, -0.517317908815, -0.510646167026, -0.506133877904, -0.501943895193, -0.500235671484, -0.499494366853, -0.498591909034, -0.50139597438, -0.500976976118, -0.506456184285, -0.50623056982, -0.513804769405, -0.516931141161, -0.524021881292, -0.529114321967, -0.535786063895, -0.540975196562, -0.549806391361, -0.55557567561, -0.562118495244, -0.571110843455, -0.578523890504, -0.588128621042, -0.591673991433, -0.603309252486, -0.608208309861, -0.619456803495, -0.623614556202, -0.634895280692, -0.639504262485, -0.648754456759, -0.653363438624, -0.659712875235, -0.664805316804, -0.671477059967, -0.676956269335, -0.68040494819, -0.686593231814, -0.690654292999, -0.697777265362, -0.699163183093, -0.706028310381, -0.708445608764, -0.714053740998, -0.714376047447, -0.717309036158, -0.71921064424], [-0.710024910386, -0.716793345845, -0.719113952322, -0.719951949094, -0.719790795876, -0.722401478154, -0.721176713661, -0.722304786221, -0.722079171739, -0.725366697573, -0.723755165329, -0.727171613748, -0.725914618561, -0.729556681513, -0.729653373454, -0.733424359014, -0.730878137988, -0.732457439676, -0.733649973565, -0.732876438082, -0.73352105098, -0.731683904154, -0.733230975168, -0.731554981578, -0.731232675104, -0.729621142786, -0.729878987971, -0.727171613711, -0.728202994377, -0.722240324934, -0.722111402363, -0.716471039402, -0.713538050689, -0.709219144247, -0.704191163629, -0.700291255632, -0.695811196034, -0.689042760769, -0.681533020716, -0.677826496737, -0.670155603587, -0.663999550742, -0.655007201422, -0.648077613287, -0.636410120856, -0.629448302266, -0.617232889248, -0.61023884021, -0.598990346709, -0.591126070533, -0.580328806276, -0.569015851931, -0.560635885853, -0.550225389661, -0.54010496934, -0.529082091324, -0.5206376644, -0.509904862377, -0.501331513109, -0.490469788818, -0.485377348365, -0.475321390163, -0.471195868845, -0.464266282357, -0.459753993514, -0.455177243418, -0.45137402858, -0.450632723992, -0.448312118361, -0.44860219404, -0.449698035625, -0.454371477572, -0.456917697711, -0.464653049979, -0.471131407592, -0.483282357051, -0.492693702657, -0.508035485456, -0.522088043056, -0.539911585558, -0.558025204138, -0.578266045382, -0.601858873674, -0.626483083273, -0.654362588553, -0.681565251366, -0.71224882486, -0.744092702944, -0.780448873256, -0.816418277644, -0.855481826546, -0.892966075707, -0.936284075784, -0.975573246475, -1.019503634723, -1.062531567617, -1.107880111461, -1.154646808241, -1.200317665994, -1.247277754457, -1.292368467699, -1.34100455941, -1.386707663505, -1.432475233028, -1.474568508417, -1.519852625568, -1.559464144987, -1.598946744905, -1.634271588084, -1.669725356739, -1.700763521852, -1.729900077529, -1.753138415857, -1.775119757793, -1.792524340144, -1.80361170409, -1.81241068786, -1.814731299025, -1.812475149306, -1.804320779705, -1.791235111838, -1.769543845466, -1.745403046532, -1.71143188441, -1.674688884542, -1.627180834679, -1.577126564795, -1.518047706938, -1.453070640671, -1.38135737042, -1.30219882384, -1.218366841609, -1.127992046752, -1.030462059294, -0.926485956427, -0.819544650698, -0.701709403981, -0.584067560439, -0.458142461785, -0.329703393025, -0.19533390736, -0.059546292283, 0.082784121787, 0.226564897832, 0.371989421375, 0.519605614793, 0.666512725505, 0.816094969741, 0.962421918486, 1.109973628512, 1.251949444581, 1.393183959693, 1.527488899303, 1.660311237483, 1.784528010615, 1.906166343397, 2.016201663976, 2.121337939531, 2.217481880751, 2.303376491683, 2.379182923551, 2.442870644673, 2.496792488978, 2.535984937287, 2.564380125067, 2.57672445783, 2.578207067045, 2.561189292331, 2.532246183905, 2.485157231178, 2.427528865298, 2.350014206541, 2.259156075714, 2.150990109623, 2.029126141282, 1.8904055732, 1.734570563254, 1.566971394115, 1.382322245342, 1.184426326374, 0.970608492196, 0.747250395204, 0.509066205683, 0.264049101386, 0.004528180618, -0.260375311122, -0.538171131096, -0.820576031503, -1.115260933764, -1.414200435406, -1.71903833033, -2.028453192339, -2.340478978614, -2.655502488952, -2.968205671777, -3.281134781401, -3.587940359215, -3.891748806981, -4.186242869138, -4.475709255059, -4.752992675415, -5.02395915739, -5.276296406007, -5.519641480332, -5.744002687703, -5.952603092839, -6.14325092322, -6.315011419137, -6.465531641869, -6.595907403787, -6.7039791576, -6.785750168332, -6.847183205524, -6.8814774191, -6.895981552919, -6.878512129785, -6.840446842986, -6.77298653917, -6.683028767301, -6.562547959387, -6.417603667947, -6.247873640808, -6.051714154371, -5.832767417038, -5.588068236284, -5.322451369195, -5.03250039276, -4.723984745866, -4.39335907776, -4.046972951256, -3.68041076967, -3.302245985531, -2.904259747987, -2.499151006579, -2.082471893594, -1.657896690003, -1.226972430874, -0.788248690179, -0.34659224316, 0.101574571531, 0.549128852274, 0.99794004534, 1.440691873864, 1.883089223901, 2.315688590355, 2.742357703593, 3.153814185862, 3.556665354349, 3.938824725544, 4.307802055414, 4.648771194708, 4.982230886135, 5.286554247973, 5.568638621824, 5.826260029219, 6.055357318603, 6.260217140354, 6.435875871716, 6.582752456123, 6.700492300534, 6.79202838416, 6.848400448848, 6.877279453822, 6.870994402281, 6.840890618981, 6.775010405327, 6.682636322387, 6.559062678139, 6.407061384714, 6.228050656109, 6.020709080125, 5.788163116111, 5.529671511214, 5.249134254804, 4.943296081938, 4.619827965986, 4.270704476852, 3.909623703226, 3.527496586161, 3.134572481773, 2.724792004513, 2.311595300989, 1.885699903608, 1.453745269663, 1.018728785616, 0.581842919588, 0.146955279198, -0.290897715685, -0.723207244305, -1.155549266911, -1.581928938196, -2.002571919715, -2.413965101174, -2.817139893542, -3.202717146175, -3.57859340424, -3.93616301468, -4.277714337744, -4.599701926599, -4.90177118411, -5.183180734068, -5.440900782798, -5.678218832441, -5.889429891994, -6.078433861212, -6.241459615534, -6.379570719093, -6.490027451168, -6.577728923312, -6.635326350273, -6.672746961474, -6.681320504889, -6.670265146349, -6.631200736434, -6.571862818298, -6.486739855383, -6.380505427068, -6.254932292263, -6.10769984155, -5.942031249561, -5.758281107182, -5.558351102183, -5.339018167199, -5.109693837164, -4.865027781983, -4.613367876412, -4.346785311362, -4.07462709678, -3.794346993999, -3.510038333336, -3.217672254619, -2.925467618447, -2.630136865355, -2.335579904363, -2.043440480452, -1.75117234287, -1.467348834592, -1.185137020595, -0.912046622996, -0.642050483247, -0.38243270481, -0.12684383114, 0.114821354973, 0.354552660666, 0.579490085203, 0.792888933492, 0.993685605466, 1.181880108564, 1.358729441583, 1.517690794561, 1.66604828599, 1.79745248593, 1.91548099088, 2.016201663979, 2.103965635885, 2.175485381126, 2.236465717242, 2.279106831693, 2.310370537258, 2.325615622902, 2.329870065433, 2.319749649111, 2.297059289292, 2.261508911229, 2.215483582179, 2.159885760796, 2.090622159789, 2.014847978107, 1.928631081568, 1.837128369633, 1.73650439991, 1.632560682816, 1.518238714889, 1.402144068285, 1.277379392366, 1.154741939, 1.024562525132, 0.895253337089, 0.763333467718, 0.630382214794, 0.498140029227, 0.366220141981, 0.235944006455, 0.106634778363, -0.017582024409, -0.142443452805, -0.262051303755, -0.38333516252, -0.494305234496, -0.607112468088, -0.710218294224, -0.814581130586, -0.906986410225, -0.997683478167, -1.082933577324, -1.162446629846, -1.237157323255, -1.303036821458, -1.367562639148, -1.422934950654, -1.475503198335, -1.519562549385, -1.56052775785, -1.593177450511, -1.624086687772, -1.641459033707, -1.659766070563, -1.670950123395, -1.677976416022, -1.679749104576, -1.675945881909, -1.670273278632, -1.657606613718, -1.643715182568, -1.624344533351, -1.60468380868, -1.580091788639, -1.554403926346, -1.522463311488, -1.491167312477, -1.45545571143, -1.420968878936, -1.38248544425, -1.345903622526, -1.305615275514, -1.267679770787, -1.227520352303, -1.186426247372, -1.148136213419, -1.10778341951, -1.068171933565, -1.029688523456, -0.991205115721, -0.951239100204, -0.917203527712, -0.879010202787, -0.848133237989, -0.812679522248, -0.784026475241, -0.752343748533, -0.724947699177, -0.697519420203, -0.672411748598, -0.648980071258, -0.626805389693, -0.606790161664, -0.585743553728, -0.570885229008, -0.554640987151, -0.544262721671, -0.530758084501, -0.52411857322, -0.513837000056, -0.510388321919, -0.501105898678, -0.497657220622, -0.495175461647, -0.492758163962, -0.492790394595, -0.491340015991, -0.494530848929, -0.496110150111, -0.500461285963, -0.503974425287, -0.511032934651, -0.516125375253, -0.524537571479, -0.527309406293, -0.536205062214, -0.543360263805, -0.551353462011, -0.558379741184, -0.565631634866, -0.574204984823, -0.582230413998, -0.589450077279, -0.597894504944, -0.608272771146, -0.615846971723, -0.625032704438, -0.63031852964, -0.638956341598, -0.642888479894, -0.652074212929, -0.65616750453, -0.664354087814, -0.669253145555, -0.676279425834, -0.680243794981, -0.684788315789, -0.691041060696, -0.694844276739, -0.698196263731, -0.702128402385, -0.704610162007, -0.704384547489, -0.707962149067, -0.709509220038, -0.7142471249, -0.713699203924]]
  in  "Open":bool
  in  "Filter lf":bool caption="Scan"
  in  "Low cutoff freq: fl":dbl=40.0
  in  "Tab Control":T7(tab)=enum."          DAQ        "
  out "Get data":bool
  out "Start Pos X":dbl
  out "Start Pos Y":dbl
  in  "Step X":dbl=1.0
  in  "Y - length":dbl=60.0
  in  "X - length":dbl=15.0
  in  "Step Y":dbl=1.0
  in  "Multiplier":dbl=10.0
  out "Cur. Pos Y":dbl format="%#_4g"
  in  "Speed (mm/s)":dbl=2.0
  in  "Travel per Pulse (mm)":dbl=0.004
  in  "COM Y":refnum<visa-resource-name>="COM3"
  in  "COM X":refnum<visa-resource-name>="COM4"
  out "Completed":bool
  out "No. X":i32
  out "No. Y":i32
  in  "Baud Rate":u32=9600
  out "Cur. Pos X":dbl format="%#_4g"
  in  "DAQ Pulser":bool=TRUE
  in  "No. Samples":dbl=2.0
  out "Sample per Channel AO":dbl=20000.0
  in  "Pulser Cycles":i32=10
  out "Actual Sample Rate":dbl=500.0 format="%0.2f"
  in  "Sensor Physical Channel":tag="Dev1/ai1:3"
  in  "Min Voltage":dbl=-10.0
  in  "Max Voltage":dbl=10.0
  in  "Terminal Configuration":i32(ring)=10083 items=["default"=-1, "RSE"=10083, "NRSE"=10078, "Differential"=10106, "Pseudodifferential"=12529]
  in  "Sample Clock Source 2":tag="OnboardClock"
  in  "Sample Rate":dbl=100000.0
  out "Actual Sample Rate 2":dbl=400000.0 format="%0.2f"
  in  "Physical Channel(s)":tag="Dev1/ao0:1"
  in  "Min Voltage 2":dbl=-10.0
  in  "Max Voltage 2":dbl=10.0
  in  "Sample Clock Source":tag="OnboardClock"
  in  "Sample Rate 2":dbl=400000.0 format="%#_6p"
  # "Pulse Shape"
  # "Trigger Settings"
  # "Data Processing"
  # "Time gate = %T/2"
  # "3D Surface"
  # "Process"
  # "Repair line"
  # "Coil Signal(0)"
  # "Hall sensor Signal(2)"
  # "Feature Extraction"
  # "Power Spectal Density"
  # "COM Setting"
  # "Speed Setting"
  # "Scan Setting"
  # "Step > S*P/f"
  # "Pulser Channel"
  # "Pulser Timming"
  # "Sensor Channel"
  # "DAQ Timming"
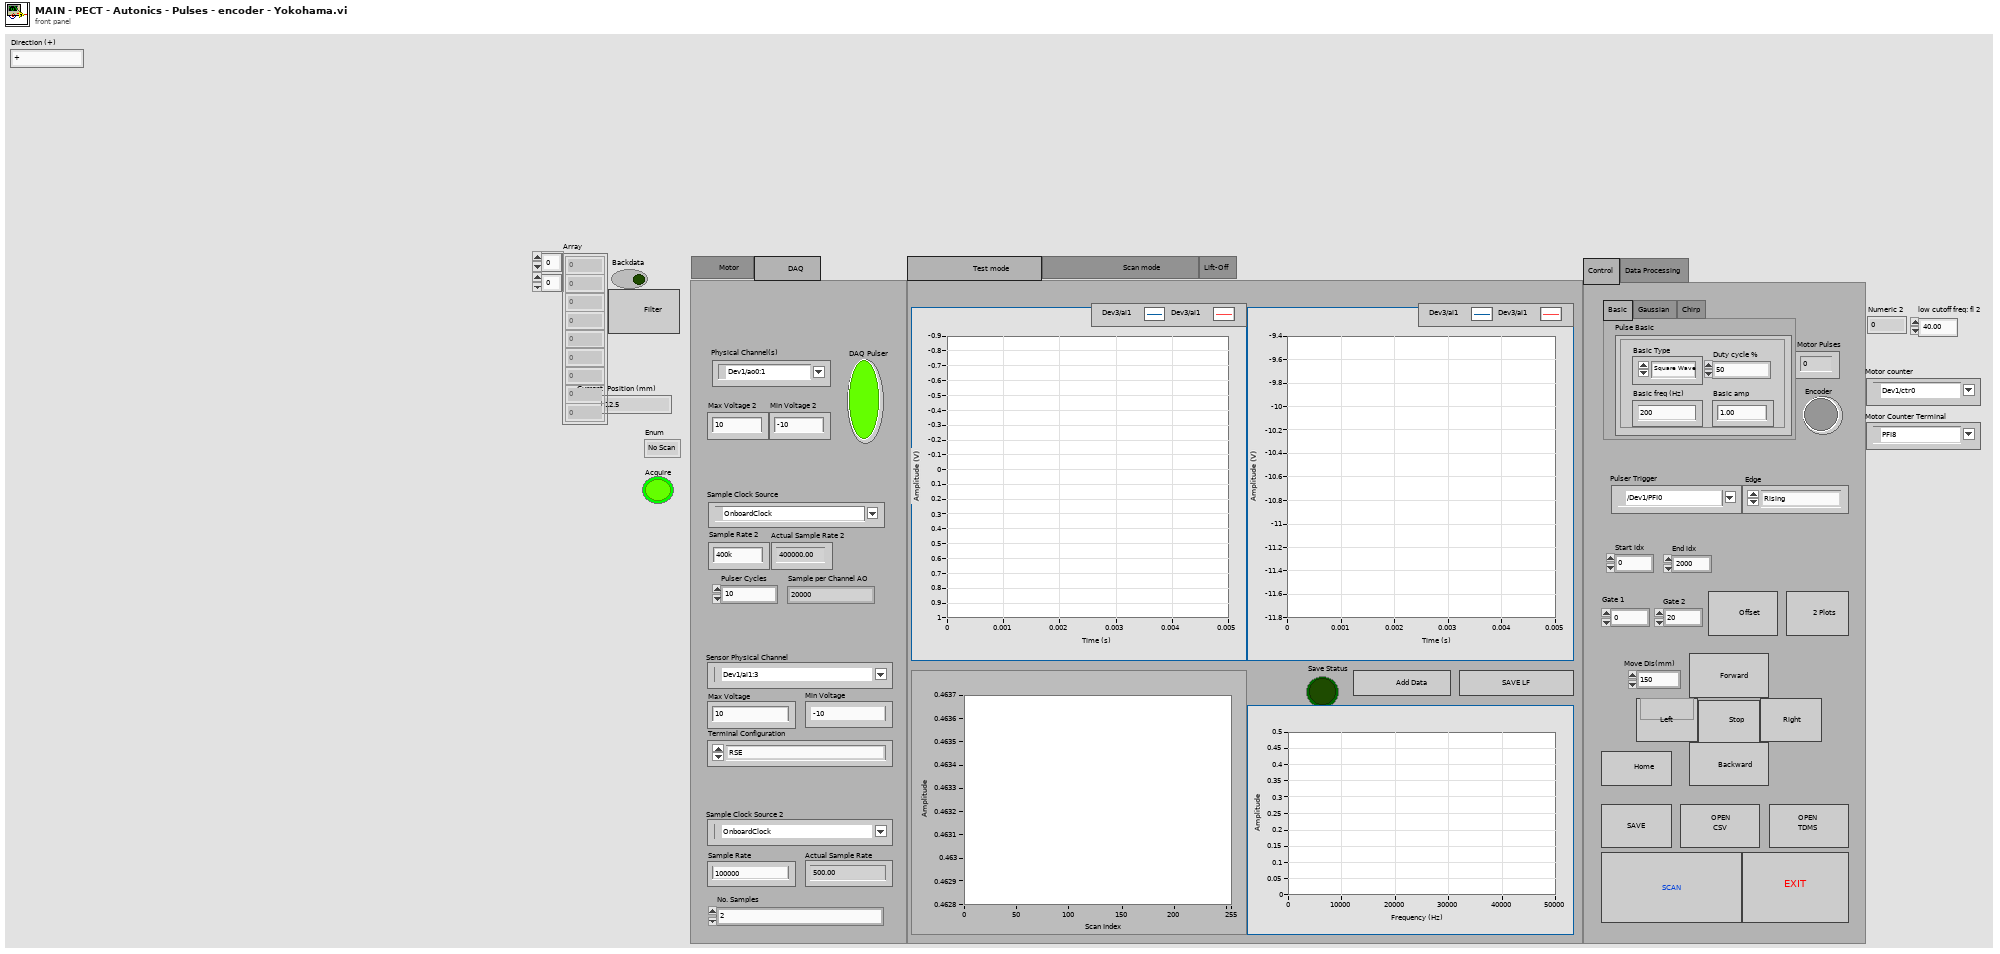
[diagram p1: front panel]
types:
  T1 = enum16{"No Scan", "Move X", "Wait X", "Move Y", "Wait Y"}
  T2 = typedef "Control 1.ctl" = dbl
  T3 = cluster{"Basic amp":T2, "Duty cycle %":dbl, "Basic freq (Hz)":u16, "Basic Type":u16}
  T4 = cluster{"Gauss amp":dbl, "Gauss Nor. Band":dbl, "Gauss atten (dB)":dbl, "Gauss freq (Hz)":dbl}
  T5 = cluster{"Chirp amp":dbl, "Chirp f2":dbl, "Chirp f1":dbl}
  T6 = enum32{"                    Test mode                   ", "                          Scan mode                      ", "Lift-Off"}
  T7 = enum32{"        Motor      ", "          DAQ        "}
  T8 = enum16{"open", "open or create", "create or replace", "create", "open (read-only)"}
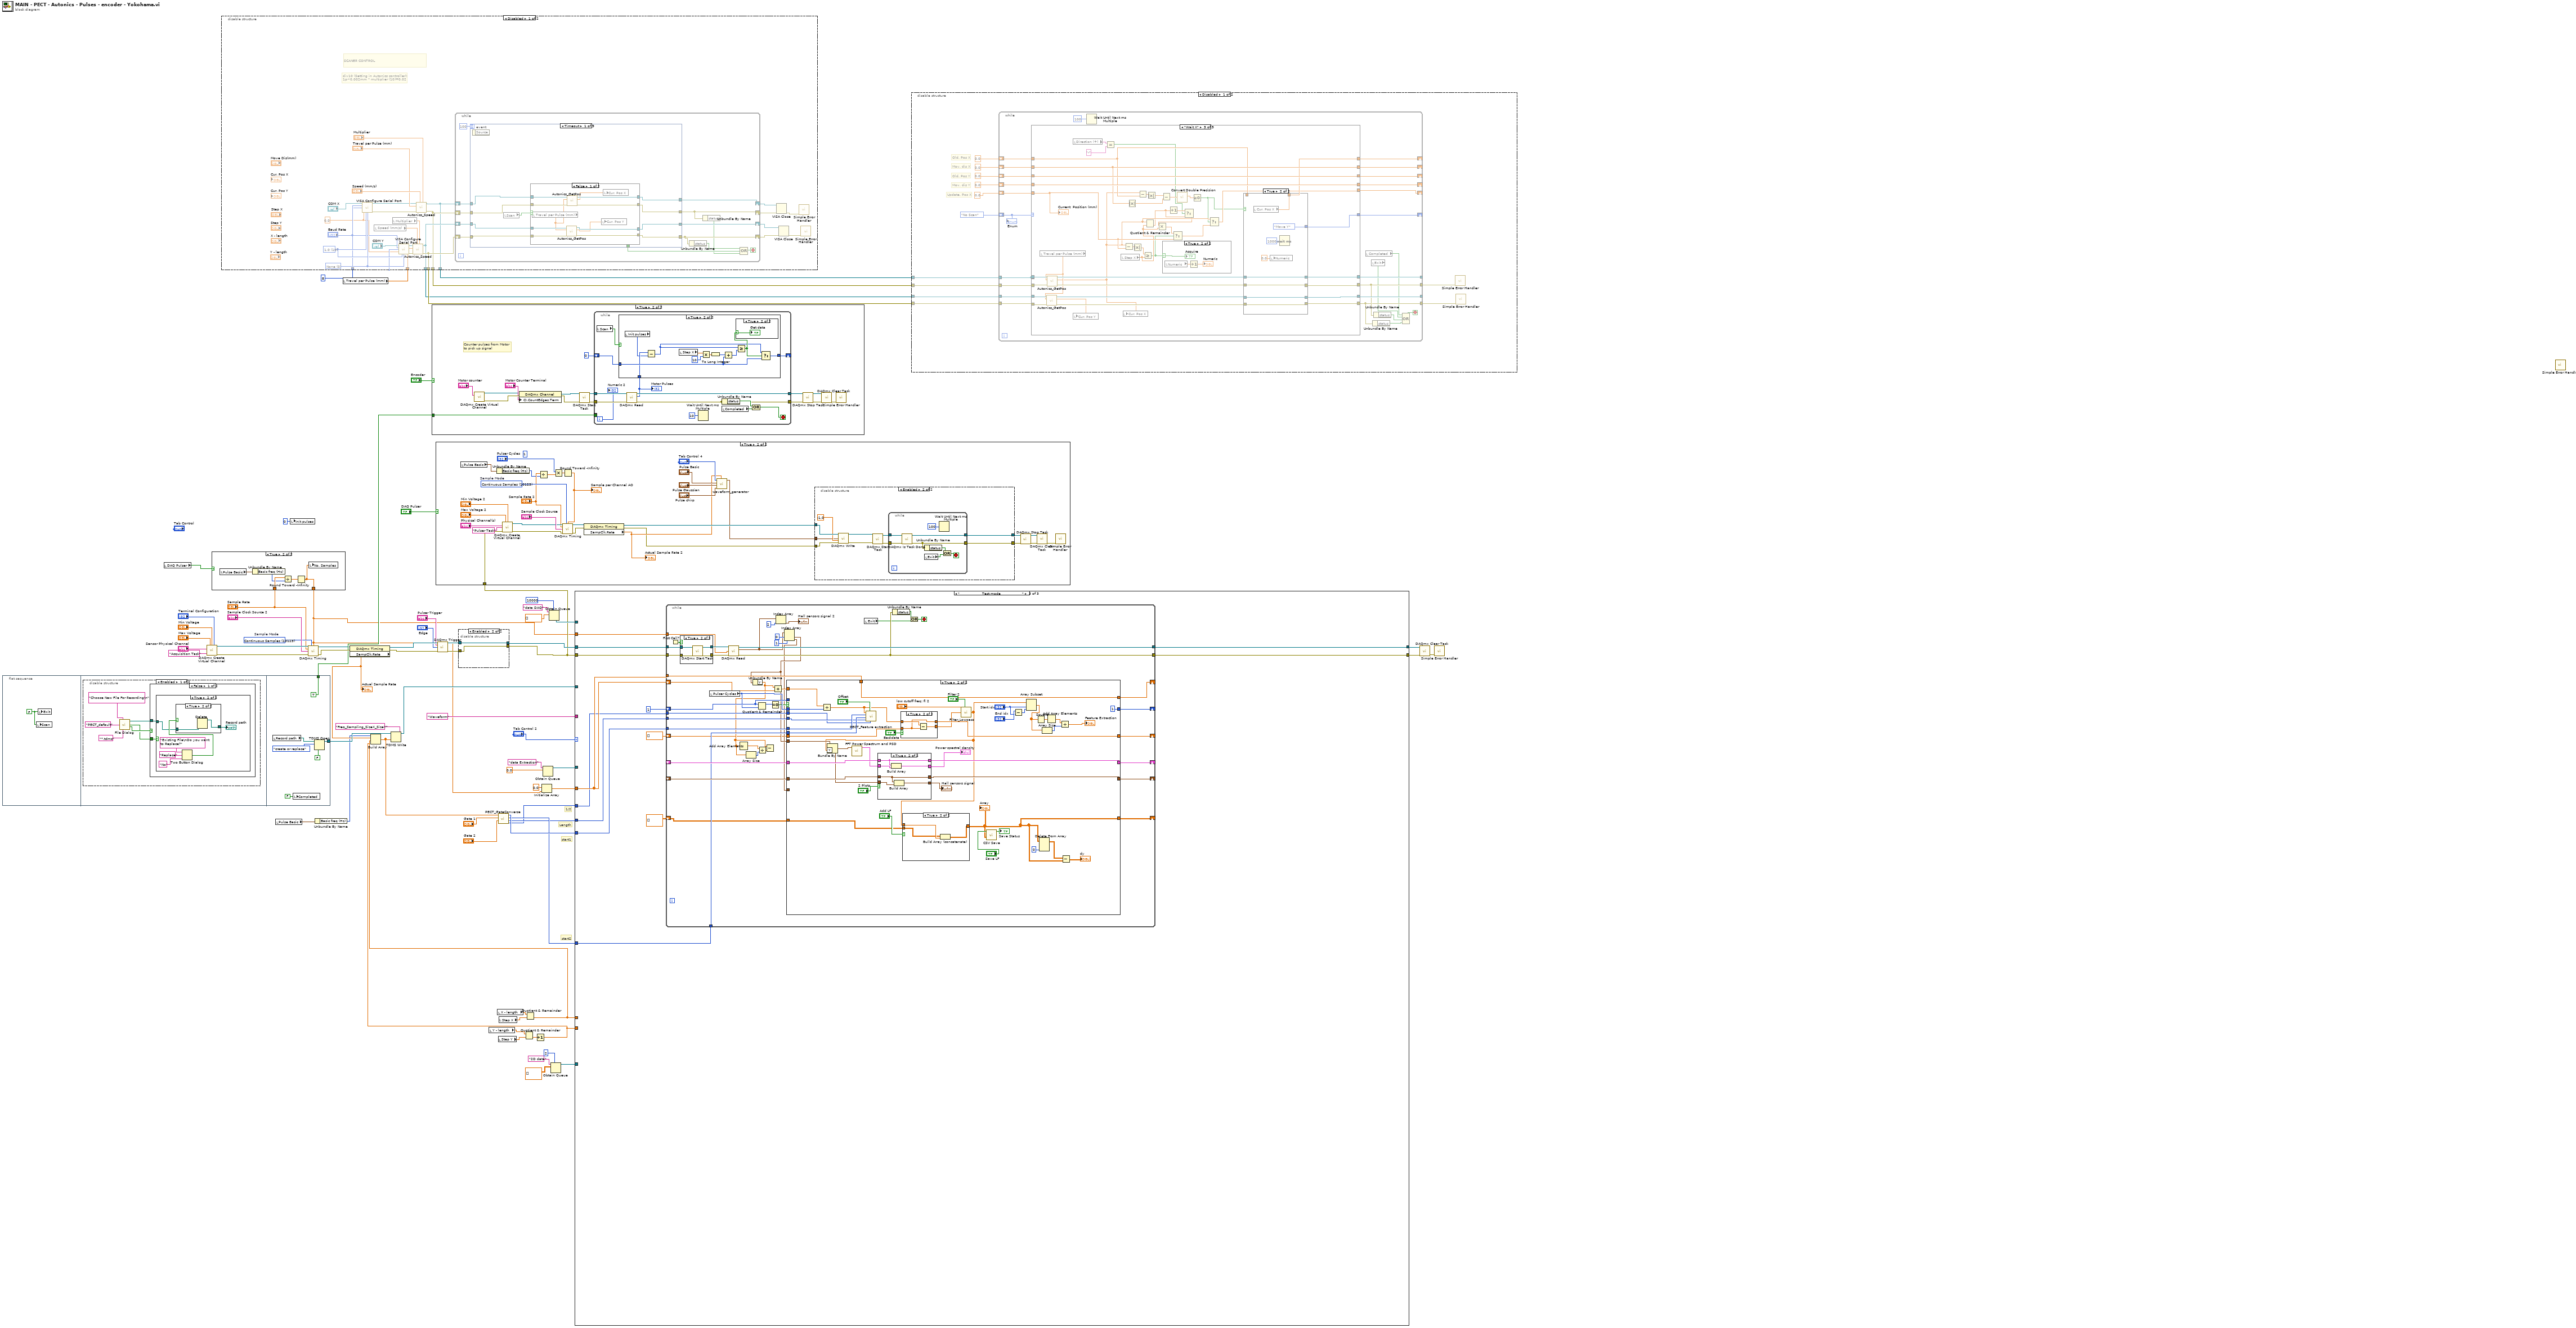
[diagram p0: block diagram]
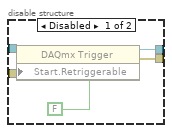
[diagram p2: hidden frame]
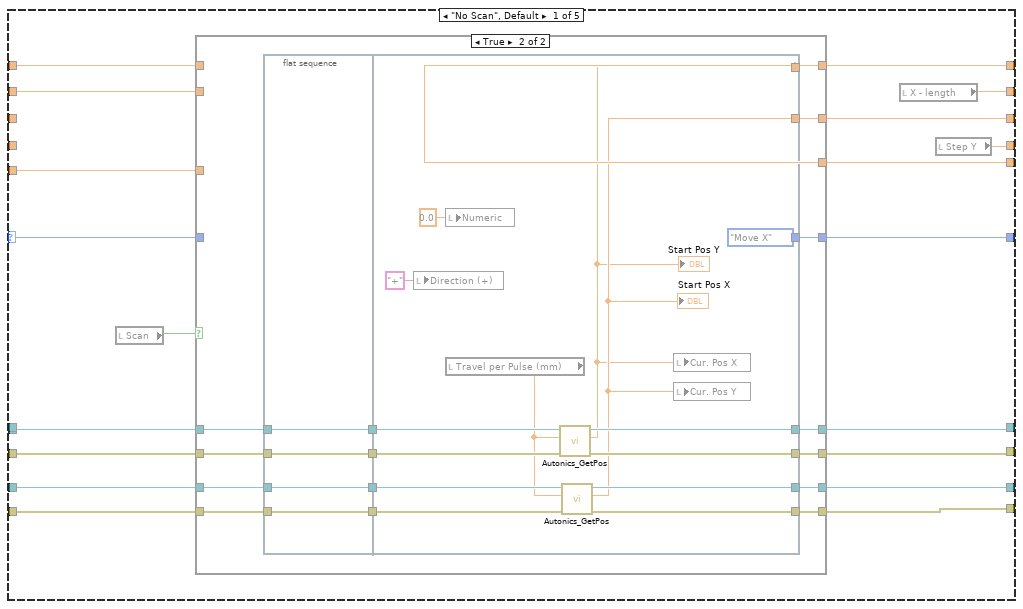
[diagram p3: hidden frame]
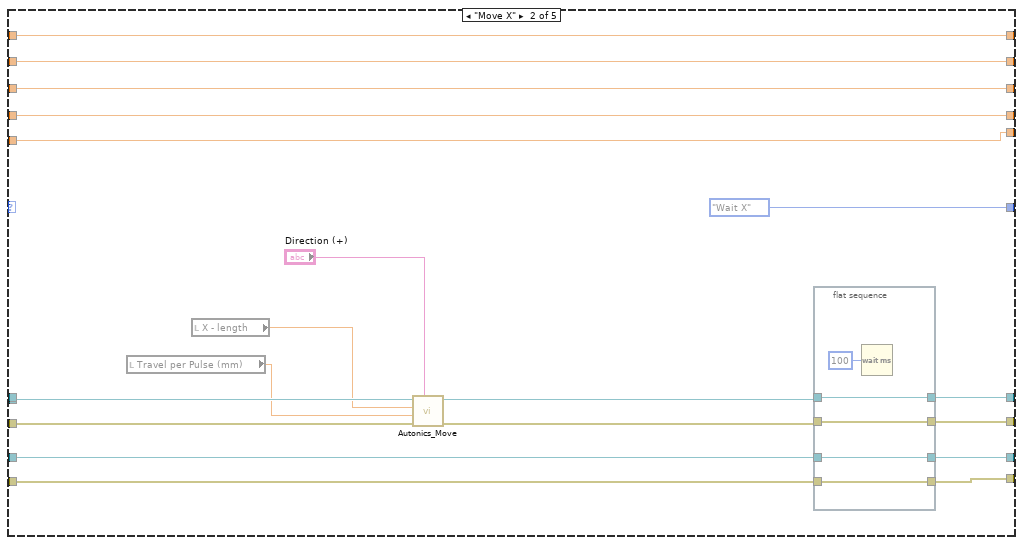
[diagram p5: hidden frame]
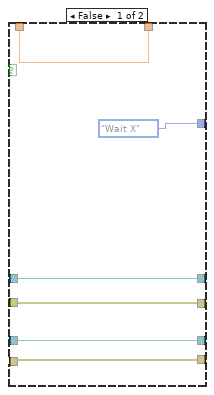
[diagram p7: hidden frame]
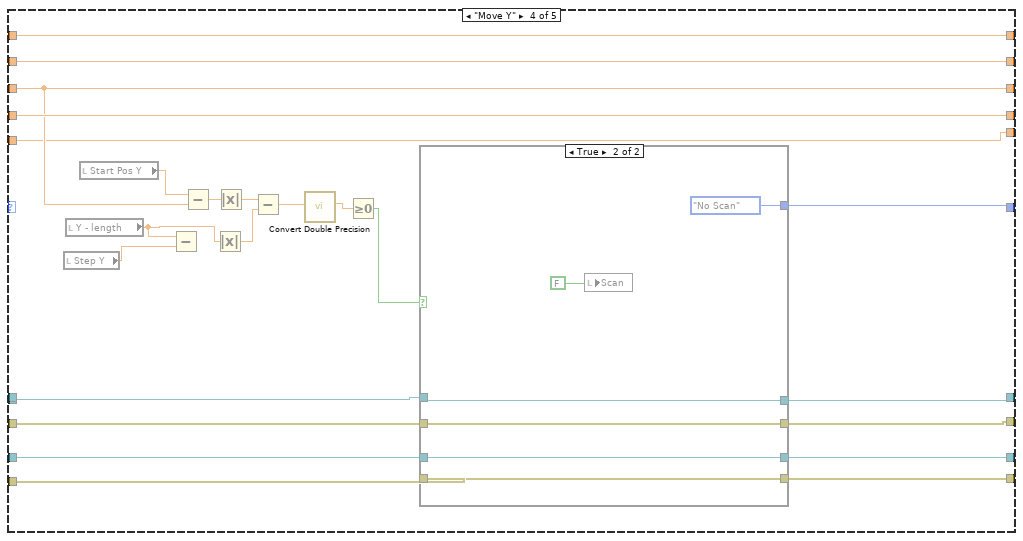
[diagram p8: hidden frame]
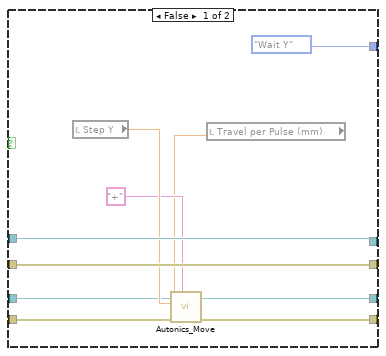
[diagram p9: hidden frame]
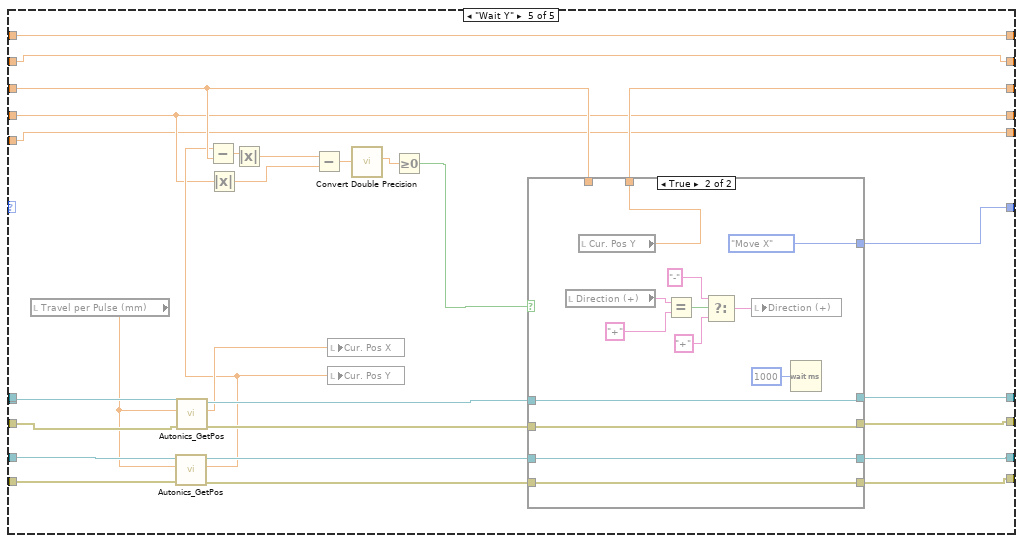
[diagram p10: hidden frame]
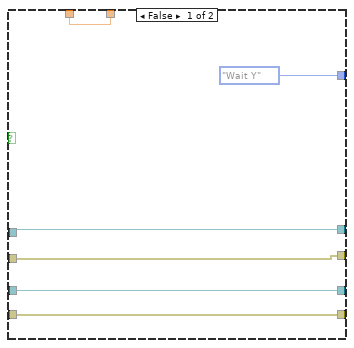
[diagram p11: hidden frame]
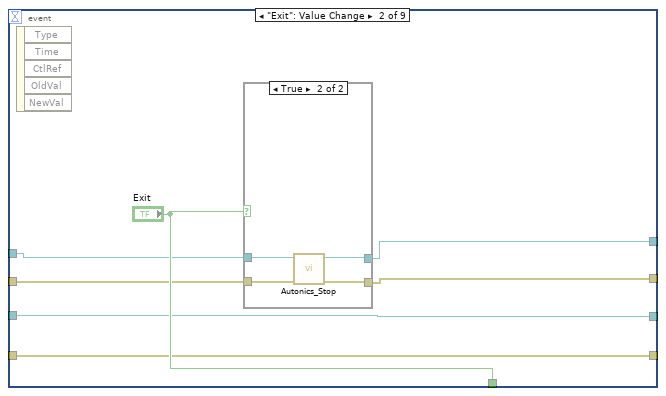
[diagram p14: hidden frame]
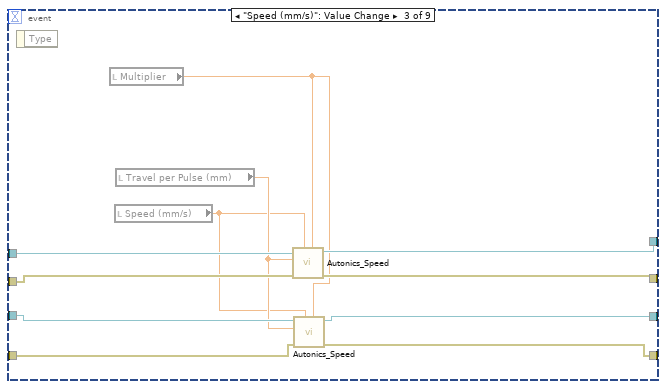
[diagram p16: hidden frame]
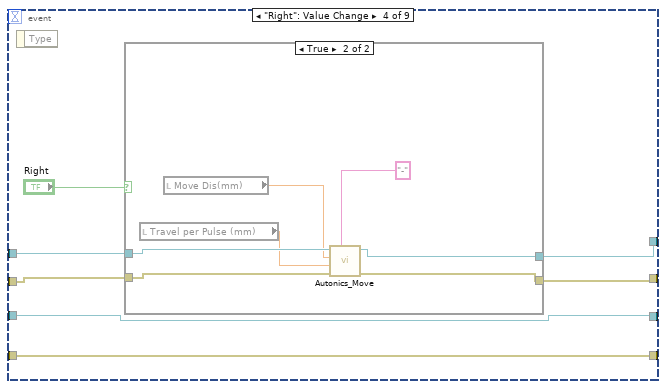
[diagram p17: hidden frame]
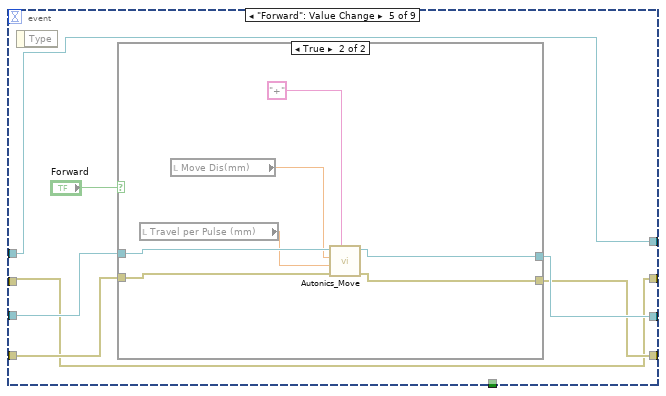
[diagram p19: hidden frame]
diagram:
  w58 = 10123 items=["Finite Samples"=10178, "Continuous Samples"=10123, "Hardware Timed Single Point"=12522]  # Sample Mode
  # "1/2"
  # "start1"
  # "start2"
  # "Length"
  n1 = flat-sequence {
    tunnel: [w95] -> w43
    tunnel: [TRUE ("disable buffering (T)")] -> w25
    frame #0 {
      w71 = FALSE ("Exit")
      n2 = local write "Scan"(w71) -> ()
      n3 = local write "Exit"(w71) -> ()
    }
    frame #1 {
      n4 = disable-structure shown="Enabled" {
        frame Enabled {
          n5 = call "File Dialog"("prompt"="Choose New File For Recording\n" ("button label"), "default name"="PECT_default", "pattern (all files)"="*.tdms") -> ("selected path"=w77:path, "exists"=w73:bool, "cancelled"=w74:bool)  [unwired: 9 in, 1 out]
          n6 = case shown="False" w74 {
            tunnel: w77 -> [w78 _]
            tunnel: w73 -> [w79 _]
            frame False {
              n7 = case shown="True" w79 {
                tunnel: w78 -> [w80 w81]
                frame False {
                  n8 = local write "Record path"(w80) -> ()
                }
                frame True {
                  n9 = Two Button Dialog(message="Existing File\nDo you want to Replace?", 1:"No" ("F button name (\"Cancel\")"), 2:"Replace" ("T button name (\"OK\")")) -> (T button?=w82:bool)
                  n10 = case shown="True" w82 {
                    tunnel: w81 -> [_ w90]
                    tunnel: [path "" ("deleted path") w89] -> w83
                    frame False {
                      n11 = local write "Exit"(TRUE ("Exit")) -> ()
                    }
                    frame True {
                      n12 = Delete(path (use dialog)=w90) -> (deleted path=w89:path)  [unwired: 4 in, 2 out]
                    }
                  }
                  "Record path" <- w83
                }
              }
            }
            frame True {
              n13 = local write "Exit"(TRUE ("Exit")) -> ()
            }
          }
        }
        frame Disabled {
        }
      }
    }
    frame #2 {
      n14 = local read "Record path"() -> (w94:path)
      n15 = local write "Completed"(FALSE ("Completed")) -> ()
      n16 = TDMS Open(6:FALSE ("disable buffering (T)"), 10:T8."create or replace" ("operation"), 11:w94) -> (3:w95:refnum<k34>)  [unwired: 4 in, 1 out]
    }
  }
  n17 = local read "DAQ Pulser"() -> (w8:bool)
  n18 = call-poly <vilib>:"DAQmx Create Virtual Channel.vi"("maximum value"="Max Voltage", "minimum value"="Min Voltage", "input terminal configuration"="Terminal Configuration", "physical channels"="Sensor Physical Channel", "name to assign"="Acquisition Task") -> ("task out"=w68:refnum<k21>, "error out"=w69:errorcluster)  [unwired: 9 in]
  n19 = case shown="True" w8 {
    tunnel: ["No. Samples" w101] -> w1
    tunnel: "Sample Rate" -> [_ w102]
    frame False {
    }
    frame True {
      n20 = local read "Pulse Basic"() -> (w100:T3)
      n21 = Unbundle By Name(w100) -> ("Basic freq (Hz)"=w99:u16)
      n22 = Divide(x=w102, y=w99) -> (x/y=w103:dbl)
      n23 = Round Toward -Infinity(1:w103) -> (0:w101:dbl)
      n24 = local write "No. Samples"(w101) -> ()
    }
  }
  n25 = local read "Pulse Basic"() -> (w10:T3)
  n26 = local write "Init pulses"(0 ("Init pulses")) -> ()
  n27 = call-poly <vilib>:"DAQmx Timing.vi"("task/channels in"=w68, "sample mode"=w58, "samples per channel"=w1, "rate"="Sample Rate", "source"="Sample Clock Source 2", "error in"=w69) -> ("task out"=w23:refnum<k21>, "error out"=w70:errorcluster)  [unwired: 8 in]
  n28 = Unbundle By Name(w10) -> ("Basic freq (Hz)"=w9:u16)
  n29 = local read "Travel per Pulse (mm)"() -> (w14:dbl)
  n30 = disable-structure shown="Disabled" {
    disable-tunnel: [w124 _] -> w19
    disable-tunnel: [w123 _] -> w18
    disable-tunnel: [w122 _] -> w17
    disable-tunnel: [w121 _] -> w16
    disable-tunnel: u16 8 ("Data bits") -> [w117 _]
    disable-tunnel: w14 -> [w115 _]
    frame Disabled {
      w116 = 0.0 ("Parity")
      w119 = u16 10 items=["1.0"=10, "1.5"=15, "2.0"=20] ("Stop bits")
      w120 = u16 0 items=["None", "XON/XOFF", "RTS/CTS", "XON/XOFF & RTS/CTS", "DTR/DSR", "XON/XOFF & DTR/DSR"] ("Flow control")
      # "div10 (Setting in Autonics controller):\n1p~0.002mm * multiplier (10)=0.02"
      # "SCANER CONTROL"
      n31 = call-poly "VISA Configure Serial Port"("VISA resource name"="COM X", "baud rate (9600)"="Baud Rate", "data bits (8)"=w117, "parity (0:none)"=w116, "stop bits (10: 1 bit)"=w119, "flow control (0:none)"=w120) -> ("VISA resource name out"=w105:refnum<visa-resource-name>, "error out"=w106:errorcluster)  [unwired: 8 in]
      n32 = local read "Speed (mm/s)"() -> (w113:dbl)
      n33 = local read "Multiplier"() -> (w114:dbl)
      n34 = call-poly "VISA Configure Serial Port"("VISA resource name"="COM Y", "baud rate (9600)"="Baud Rate", "data bits (8)"=w117, "parity (0:none)"=w116, "stop bits (10: 1 bit)"=w119, "flow control (0:none)"=w120) -> ("VISA resource name out"=w110:refnum<visa-resource-name>, "error out"=w111:errorcluster)  [unwired: 8 in]
      n35 = call "Autonics_Speed.vi"("Multiplier"=w114, "Speed (mm/s)"=w113, "error in (no error)"=w111, "Travel per  Pulse"=w115, "VISA resource name"=w110) -> ("error out"=w124:errorcluster, "VISA resource name out"=w123:refnum<visa-resource-name>)  [unwired: 5 in]
      n36 = call "Autonics_Speed.vi"("Multiplier"="Multiplier", "Speed (mm/s)"="Speed (mm/s)", "error in (no error)"=w106, "Travel per  Pulse"="Travel per Pulse (mm)", "VISA resource name"=w105) -> ("error out"=w122:errorcluster, "VISA resource name out"=w121:refnum<visa-resource-name>)  [unwired: 5 in]
      n37 = while {
        shift-right: [w143] -> w128
        shift-left: w121 -> [w142]
        shift-right: [w133] -> w127
        shift-left: w122 -> [w141]
        shift-right: [w136] -> w129
        shift-left: w123 -> [w138]
        shift-right: [w135] -> w130
        shift-left: w124 -> [w137]
        stop <- w140 stop-if-true
        n38 = event shown="[0] Timeout" {
          selector: _ -> [_ _ _ _ _ _ _ _ _]
          dyn-events: _ -> [_ _ _ _ _ _ _ _ _]
          timeout: 100 -> [_ _ _ _ _ _ _ _ _]
          tunnel: w142 -> [w151 w173 w191 w196 w208 w228 w241 w264 w291]
          tunnel: w141 -> [w150 w172 w190 w195 w209 w227 w240 w263 w290]
          tunnel: [w147 w171 w189 w198 w208 w230 w241 w261 w293] -> w143
          tunnel: [w146 w170 w188 w197 w209 w229 w240 w260 w292] -> w133
          tunnel: [_ "Exit" _ _ _ _ _ _ _] -> w139
          tunnel: w138 -> [w149 w168 w187 w193 w213 w225 w244 w259 w288]
          tunnel: w137 -> [w148 w169 w184 w192 w212 w224 w245 w258 w286]
          tunnel: [w145 w168 w186 w193 w211 w225 w242 w256 w287] -> w136
          tunnel: [w144 w169 w185 w192 w210 w224 w243 w257 w285] -> w135
          event Timeout {
            n39 = event-data() -> ()  [unwired: 1 in, 1 out]
            n40 = local read "Scan"() -> (w152:bool)
            n41 = case shown="False" w152 {
              tunnel: w149 -> [w163 w165]
              tunnel: w148 -> [w162 w164]
              tunnel: [w161 w165] -> w145
              tunnel: [w160 w164] -> w144
              tunnel: w150 -> [w159 w166]
              tunnel: w151 -> [w158 w167]
              tunnel: [w157 w167] -> w147
              tunnel: [w156 w166] -> w146
              frame False {
                n42 = local read "Travel per Pulse (mm)"() -> (w155:dbl)
                n43 = call "Autonics_GetPos.vi"("error in (no error)"=w162, "Travel per Pulse (mm)"=w155, "VISA resource name"=w163) -> ("error out"=w160:errorcluster, "Current  Position (mm)"=w153:dbl, "VISA resource name out"=w161:refnum<visa-resource-name>)  [unwired: 6 in]
                n44 = call "Autonics_GetPos.vi"("error in (no error)"=w159, "Travel per Pulse (mm)"=w155, "VISA resource name"=w158) -> ("error out"=w156:errorcluster, "Current  Position (mm)"=w154:dbl, "VISA resource name out"=w157:refnum<visa-resource-name>)  [unwired: 6 in]
                n45 = local write "Cur. Pos Y"(w153) -> ()
                n46 = local write "Cur. Pos X"(w154) -> ()
              }
              frame True {
              }
            }
          }
          event "Exit": Value Change {
            n47 = event-data() -> ()  [unwired: 1 in, 5 out]
            n48 = case shown="True" "Exit" {
              tunnel: [w176 w179] -> w171
              tunnel: [w175 w180] -> w170
              tunnel: w173 -> [w176 w178]
              tunnel: w172 -> [w175 w177]
              frame False {
              }
              frame True {
                n49 = call "Autonics_Stop.vi"("error in (no error)"=w177, "VISA resource name"=w178) -> ("error out"=w180:errorcluster, "VISA resource name out"=w179:refnum<visa-resource-name>)  [unwired: 8 in]
              }
            }
          }
          event "Speed (mm/s)": Value Change {
            n50 = event-data() -> ()  [unwired: 1 in, 1 out]
            n51 = local read "Multiplier"() -> (w181:dbl)
            n52 = local read "Speed (mm/s)"() -> (w182:dbl)
            n53 = local read "Travel per Pulse (mm)"() -> (w183:dbl)
            n54 = call "Autonics_Speed.vi"("Multiplier"=w181, "Speed (mm/s)"=w182, "error in (no error)"=w190, "Travel per  Pulse"=w183, "VISA resource name"=w191) -> ("error out"=w188:errorcluster, "VISA resource name out"=w189:refnum<visa-resource-name>)  [unwired: 5 in]
            n55 = call "Autonics_Speed.vi"("Multiplier"=w181, "Speed (mm/s)"=w182, "error in (no error)"=w184, "Travel per  Pulse"=w183, "VISA resource name"=w187) -> ("error out"=w185:errorcluster, "VISA resource name out"=w186:refnum<visa-resource-name>)  [unwired: 5 in]
          }
          event "Right": Value Change {
            n56 = event-data() -> ()  [unwired: 1 in, 1 out]
            n57 = case shown="True" "Right" {
              tunnel: [w199 w205] -> w198
              tunnel: [w200 w201] -> w197
              tunnel: w196 -> [w199 w207]
              tunnel: w195 -> [w200 w206]
              frame False {
              }
              frame True {
                n58 = local read "Travel per Pulse (mm)"() -> (w203:dbl)
                n59 = local read "Move Dis(mm)"() -> (w204:dbl)
                n60 = call "Autonics_Move.vi"("Direction (+)"="-", "error in (no error)"=w206, "Travel per Pulse (mm)"=w203, "Move Distance (mm)"=w204, "VISA resource name"=w207) -> ("error out"=w201:errorcluster, "VISA resource name out"=w205:refnum<visa-resource-name>)  [unwired: 5 in]
              }
            }
          }
          event "Forward": Value Change {
            n61 = event-data() -> ()  [unwired: 1 in, 1 out]
            n62 = case shown="True" "Forward" {
              tunnel: [w215 w221] -> w211
              tunnel: [w216 w220] -> w210
              tunnel: w213 -> [w215 w223]
              tunnel: w212 -> [w216 w222]
              frame False {
              }
              frame True {
                n63 = local read "Travel per Pulse (mm)"() -> (w218:dbl)
                n64 = local read "Move Dis(mm)"() -> (w219:dbl)
                n65 = call "Autonics_Move.vi"("Direction (+)"="+", "error in (no error)"=w222, "Travel per Pulse (mm)"=w218, "Move Distance (mm)"=w219, "VISA resource name"=w223) -> ("error out"=w220:errorcluster, "VISA resource name out"=w221:refnum<visa-resource-name>)  [unwired: 5 in]
              }
            }
          }
          event "Left": Value Change {
            n66 = event-data() -> ()  [unwired: 1 in, 1 out]
            n67 = case shown="True" "Left" {
              tunnel: [w232 w237] -> w230
              tunnel: [w231 w236] -> w229
              tunnel: w228 -> [w232 w239]
              tunnel: w227 -> [w231 w238]
              frame False {
              }
              frame True {
                # "Moving distance"
                n68 = local read "Travel per Pulse (mm)"() -> (w233:dbl)
                n69 = local read "Move Dis(mm)"() -> (w234:dbl)
                n70 = call "Autonics_Move.vi"("Direction (+)"="+", "error in (no error)"=w238, "Travel per Pulse (mm)"=w233, "Move Distance (mm)"=w234, "VISA resource name"=w239) -> ("error out"=w236:errorcluster, "VISA resource name out"=w237:refnum<visa-resource-name>)  [unwired: 5 in]
              }
            }
          }
          event "Backward": Value Change {
            n71 = event-data() -> ()  [unwired: 1 in, 1 out]
            n72 = case shown="True" "Backward" {
              tunnel: [w248 w253] -> w242
              tunnel: [w247 w252] -> w243
              tunnel: w244 -> [w248 w255]
              tunnel: w245 -> [w247 w254]
              frame False {
              }
              frame True {
                # "Moving distance"
                n73 = local read "Travel per Pulse (mm)"() -> (w249:dbl)
                n74 = local read "Move Dis(mm)"() -> (w250:dbl)
                n75 = call "Autonics_Move.vi"("Direction (+)"="-", "error in (no error)"=w254, "Travel per Pulse (mm)"=w249, "Move Distance (mm)"=w250, "VISA resource name"=w255) -> ("error out"=w252:errorcluster, "VISA resource name out"=w253:refnum<visa-resource-name>)  [unwired: 5 in]
              }
            }
          }
          event "Home": Value Change {
            n76 = event-data() -> ()  [unwired: 1 in, 1 out]
            n77 = case shown="True" "Home" {
              tunnel: [w268 w280] -> w261
              tunnel: [w267 w279] -> w260
              tunnel: w264 -> [w268 w284]
              tunnel: w263 -> [w267 w283]
              tunnel: w259 -> [w266 w276]
              tunnel: w258 -> [w265 w275]
              tunnel: [w266 w274] -> w256
              tunnel: [w265 w273] -> w257
              frame False {
              }
              frame True {
                n78 = call "Autonics_Home.vi"("error in (no error)"=w283, "VISA resource name"=w284) -> ("error out"=w281:errorcluster, "VISA resource name out"=w282:refnum<visa-resource-name>)  [unwired: 8 in]
                n79 = call "Autonics_Home.vi"("error in (no error)"=w275, "VISA resource name"=w276) -> ("error out"=w278:errorcluster, "VISA resource name out"=w277:refnum<visa-resource-name>)  [unwired: 8 in]
                n80 = local read "Travel per Pulse (mm)"() -> (w272:dbl)
                n81 = local read "Speed (mm/s)"() -> (w271:dbl)
                n82 = local read "Multiplier"() -> (w270:dbl)
                n83 = local write "Home"(FALSE ("Home")) -> ()
                n84 = call "Autonics_Speed.vi"("Multiplier"=w270, "Speed (mm/s)"=w271, "error in (no error)"=w281, "Travel per  Pulse"=w272, "VISA resource name"=w282) -> ("error out"=w279:errorcluster, "VISA resource name out"=w280:refnum<visa-resource-name>)  [unwired: 5 in]
                n85 = call "Autonics_Speed.vi"("Multiplier"=w270, "Speed (mm/s)"=w271, "error in (no error)"=w278, "Travel per  Pulse"=w272, "VISA resource name"=w277) -> ("error out"=w273:errorcluster, "VISA resource name out"=w274:refnum<visa-resource-name>)  [unwired: 5 in]
              }
            }
          }
          event "Stop": Value Change {
            n86 = event-data() -> ()  [unwired: 1 in, 1 out]
            n87 = case shown="False" "Stop" {
              tunnel: [w295 w302] -> w293
              tunnel: [w297 w305] -> w292
              tunnel: w291 -> [w295 w304]
              tunnel: w290 -> [w297 w303]
              tunnel: w288 -> [w296 w301]
              tunnel: [w296 w300] -> w287
              tunnel: w286 -> [w294 w299]
              tunnel: [w294 w298] -> w285
              frame False {
              }
              frame True {
                n88 = call "Autonics_Stop.vi"("error in (no error)"=w303, "VISA resource name"=w304) -> ("error out"=w305:errorcluster, "VISA resource name out"=w302:refnum<visa-resource-name>)  [unwired: 8 in]
                n89 = call "Autonics_Stop.vi"("error in (no error)"=w299, "VISA resource name"=w301) -> ("error out"=w298:errorcluster, "VISA resource name out"=w300:refnum<visa-resource-name>)  [unwired: 8 in]
              }
            }
          }
        }
        n90 = Unbundle By Name(w135) -> ("status"=w134:bool)
        n91 = Unbundle By Name(w133) -> ("status"=w132:bool)
        n92 = Compound Arithmetic op=OR(w134, w139, w132) -> (w140:bool)
      }
      n93 = VISA Close(VISA resource name=w128, error in (no error)=w127) -> (error out=w125:errorcluster)
      n94 = VISA Close(VISA resource name=w129, error in (no error)=w130) -> (error out=w126:errorcluster)
      n95 = call <vilib>:"Simple Error Handler.vi"("error in (no error)"=w125) -> ()  [unwired: 4 in, 5 out]
      n96 = call <vilib>:"Simple Error Handler.vi"("error in (no error)"=w126) -> ()  [unwired: 4 in, 5 out]
    }
    frame Enabled {
    }
  }
  n97 = property class="DAQmx Timing"(reference=w23, error in=w70) -> (reference out=w21:refnum<k21>, error out=w20:errorcluster, "SampClk.Rate"=w27:dbl)
  "Actual Sample Rate" <- w27
  n98 = case shown="True" "Encoder" {
    tunnel: w25 -> [_ w320]
    frame False {
    }
    frame True {
      # "Counter pulses from Motor\nto pick up signal"
      n99 = call-poly <vilib>:"DAQmx Create Virtual Channel.vi"("counter"="Motor counter") -> ("task out"=w313:refnum<k21>, "error out"=w315:errorcluster)  [unwired: 13 in]
      n100 = property class="DAQmx Channel"(reference=w313, error in=w315, "CI.CountEdges.Term"="Motor Counter Terminal") -> (reference out=w308:refnum<k21>, error out=w309:errorcluster)
      n101 = call <vilib>:"DAQmx Start Task.vi"("task/channels in"=w308, "error in"=w309) -> ("task out"=w310:refnum<k21>, "error out"=w307:errorcluster)  [unwired: 12 in]
      n102 = while {
        tunnel: w310 -> [w334]
        tunnel: w307 -> [w333]
        tunnel: [w327] -> w317
        tunnel: [w332] -> w316
        tunnel: [w326] -> _
        tunnel: w320 -> [w326]
        shift-right: [w325] -> _
        shift-left: u32 0 ("data") -> [w324]
        i -> [w321]
        stop <- w328 stop-if-true
        n103 = local read "Scan"() -> (w322:bool)
        n104 = call-poly <vilib>:"DAQmx Read.vi"("task/channels in"=w334, "error in"=w333) -> ("task out"=w332:refnum<k21>, "data"=w323:u32, "error out"=w327:errorcluster)  [unwired: 11 in]
        "Motor Pulses" <- w323
        n105 = case shown="True" w322 {
          tunnel: [w335 w346] -> w325
          tunnel: w324 -> [w335 w345]
          tunnel: w323 -> [_ w338]
          frame False {
          }
          frame True {
            n106 = local read "Init pulses"() -> (w337:i32)
            n107 = Subtract(x=w338, y=w337) -> (x-y=w336:u32)
            n108 = local read "Step X"() -> (w344:dbl)
            n109 = Multiply(x=w344, y=10) -> (x*y=w342:dbl)
            n110 = To Long Integer(number=w342) -> (32bit integer=w341:i32)
            n111 = Add(x=w341, y=w345) -> (x+y=w340:u32)
            n112 = Greater Or Equal?(x=w336, y=w340) -> (x >= y?=w339:bool)
            n113 = case shown="True" w339 {
              selector: w339 -> [_ w347]
              frame False {
              }
              frame True {
                "Get data" <- w347
              }
            }
            n114 = Select(t=w336, s=w339, f=w345) -> (s? t:f=w346:u32)
          }
        }
        n115 = Wait Until Next ms Multiple(millisecond multiple=u32 10 ("milliseconds to wait")) -> ()  [unwired: 1 out]
        n116 = local read "Completed"() -> (w329:bool)
        n117 = Unbundle By Name(w327) -> ("status"=w330:bool)
        n118 = Compound Arithmetic op=OR(w330, w329) -> (w328:bool)
        "Numeric 2" <- w321
      }
      n119 = call <vilib>:"DAQmx Stop Task.vi"("task/channels in"=w316, "error in"=w317) -> ("task out"=w319:refnum<k21>, "error out"=w318:errorcluster)  [unwired: 12 in]
      n120 = call <vilib>:"DAQmx Clear Task.vi"("task in"=w319, "error in"=w318) -> ("error out"=w311:errorcluster)  [unwired: 13 in]
      n121 = call <vilib>:"Simple Error Handler.vi"("error in (no error)"=w311) -> ()  [unwired: 4 in, 5 out]
    }
  }
  n122 = call-poly <vilib>:"DAQmx Trigger.vi"("task/channels in"=w21, "source"="Pulser Trigger", "edge"="Edge", "error in"=w20) -> ("task out"=w5:refnum<k21>, "error out"=w4:errorcluster)  [unwired: 10 in]
  n123 = disable-structure shown="Enabled" {
    disable-tunnel: [w352 w354] -> w45
    disable-tunnel: [w351 w353] -> w26
    disable-tunnel: w5 -> [w350 w354]
    disable-tunnel: w4 -> [w349 w353]
    frame Disabled {
      n124 = property class="DAQmx Trigger"(reference=w350, error in=w349, "Start.Retriggerable"=FALSE) -> (reference out=w352:refnum<k21>, error out=w351:errorcluster)
    }
    frame Enabled {
    }
  }
  n125 = case shown="True" "DAQ Pulser" {
    tunnel: w26 -> [_ w385]
    frame False {
    }
    frame True {
      (unwired) 1 ("x")
      w382 = 10123 items=["Finite Samples"=10178, "Continuous Samples"=10123, "Hardware Timed Single Point"=12522]  # Sample Mode
      n126 = local read "Pulse Basic"() -> (w356:T3)
      n127 = Unbundle By Name(w356) -> ("Basic freq (Hz)"=w355:u16)
      n128 = call-poly <vilib>:"DAQmx Create Virtual Channel.vi"("maximum value"="Max Voltage 2", "minimum value"="Min Voltage 2", "physical channels"="Physical Channel(s)", "name to assign"="Pulser Task", "error in"=w385) -> ("task out"=w376:refnum<k21>, "error out"=w375:errorcluster)  [unwired: 9 in]
      n129 = Divide(x="Sample Rate 2", y=w355) -> (x/y=w373:dbl)
      n130 = Multiply(x="Pulser Cycles", y=w373) -> (x*y=w372:dbl)
      n131 = Round Toward -Infinity(1:w372) -> (0:w364:dbl)
      "Sample per Channel AO" <- w364
      n132 = call-poly <vilib>:"DAQmx Timing.vi"("task/channels in"=w376, "sample mode"=w382, "samples per channel"=w364, "rate"="Sample Rate 2", "source"="Sample Clock Source", "error in"=w375) -> ("task out"=w384:refnum<k21>, "error out"=w383:errorcluster)  [unwired: 8 in]
      n133 = property class="DAQmx Timing"(reference=w384, error in=w383) -> (reference out=w371:refnum<k21>, error out=w357:errorcluster, "SampClk.Rate"=w359:dbl)
      "Actual Sample Rate 2" <- w359
      n134 = call "waveform_generator.vi"("Sampling rate"=w359, "Pulse chirp"="Pulse chirp", "Pulse Gaussian"="Pulse Gaussian", "Cluster Basic"="Pulse Basic", "Tab Control"="Tab Control 4") -> ("Waveform Graph"=w358:waveform(dbl)[])  [unwired: 6 in]
      n135 = disable-structure shown="Enabled" {
        disable-tunnel: w358 -> [w390 w411]
        disable-tunnel: [w389 w414] -> w368
        disable-tunnel: [w388 w413] -> w365
        disable-tunnel: w371 -> [w387 w415]
        disable-tunnel: w357 -> [w386 w410]
        frame Disabled {
          n136 = while {
            tunnel: w390 -> [w401]
            shift-right: [w397] -> w389
            shift-left: w387 -> [w395]
            shift-right: [w396] -> w388
            shift-left: w386 -> [w394]
            stop <- FALSE stop-if-true
            n137 = call-poly <vilib>:"DAQmx Write.vi"("task/channels in"=w395, "data"=w401, "timeout"=-1.0, "error in"=w394) -> ("task out"=w400:refnum<k21>, "error out"=w399:errorcluster)  [unwired: 9 in, 1 out]
            n138 = call <vilib>:"DAQmx Start Task.vi"("task/channels in"=w400, "error in"=w399) -> ("task out"=w393:refnum<k21>, "error out"=w392:errorcluster)  [unwired: 12 in]
            n139 = disable-structure shown="Enabled" {
              disable-tunnel: [w407 w409] -> w397
              disable-tunnel: [w406 w408] -> w396
              disable-tunnel: w393 -> [w405 w409]
              disable-tunnel: w392 -> [w404 w408]
              frame Disabled {
                n140 = call <vilib>:"DAQmx Wait Until Done.vi"("task/channels in"=w405, "error in"=w404) -> ("task out"=w403:refnum<k21>, "error out"=w402:errorcluster)  [unwired: 12 in]
                n141 = call <vilib>:"DAQmx Stop Task.vi"("task/channels in"=w403, "error in"=w402) -> ("task out"=w407:refnum<k21>, "error out"=w406:errorcluster)  [unwired: 12 in]
              }
              frame Enabled {
              }
            }
          }
        }
        frame Enabled {
          n142 = call-poly <vilib>:"DAQmx Write.vi"("task/channels in"=w415, "data"=w411, "timeout"=-1.0, "error in"=w410) -> ("task out"=w417:refnum<k21>, "error out"=w419:errorcluster)  [unwired: 9 in, 1 out]
          n143 = call <vilib>:"DAQmx Start Task.vi"("task/channels in"=w417, "error in"=w419) -> ("task out"=w416:refnum<k21>, "error out"=w418:errorcluster)  [unwired: 12 in]
          n144 = while {
            tunnel: w416 -> [w427]
            tunnel: w418 -> [w426]
            tunnel: [w424] -> w413
            tunnel: [w425] -> w414
            stop <- w421 stop-if-true
            n145 = call <vilib>:"DAQmx Is Task Done.vi"("task/channels in"=w427, "error in"=w426) -> ("task out"=w425:refnum<k21>, "error out"=w424:errorcluster)  [unwired: 11 in, 1 out]
            n146 = Unbundle By Name(w424) -> ("status"=w422:bool)
            n147 = local read "Exit"() -> (w420:bool)
            n148 = Wait Until Next ms Multiple(millisecond multiple=u32 100) -> ()  [unwired: 1 out]
            n149 = Compound Arithmetic op=OR(w422, w420) -> (w421:bool)
          }
        }
      }
      n150 = call <vilib>:"DAQmx Stop Task.vi"("task/channels in"=w368, "error in"=w365) -> ("task out"=w367:refnum<k21>, "error out"=w366:errorcluster)  [unwired: 12 in]
      n151 = call <vilib>:"DAQmx Clear Task.vi"("task in"=w367, "error in"=w366) -> ("error out"=w381:errorcluster)  [unwired: 13 in]
      n152 = call <vilib>:"Simple Error Handler.vi"("error in (no error)"=w381) -> ()  [unwired: 4 in, 5 out]
    }
  }
  n153 = local read "Y - length"() -> (w13:dbl)
  n154 = local read "X - length"() -> (w49:dbl)
  n155 = local read "Step Y"() -> (w47:dbl)
  n156 = local read "Step X"() -> (w48:dbl)
  n157 = Quotient & Remainder(x=w13, y=w47) -> (floor(x/y)=w24:dbl)  [unwired: 1 out]
  n158 = Quotient & Remainder(x=w49, y=w48) -> (floor(x/y)=w41:dbl)  [unwired: 1 out]
  n159 = Increment(x=w24) -> (x+1=w12:dbl)
  n160 = Build Array(w9, w27, w41, w12) -> (w32:dbl[])
  n161 = TDMS Write(0:w43, 5:"Freq_Sampling_SizeX_SizeY" ("group name in (Untitled)"), 9:w32) -> (4:w42:refnum<k34>)  [unwired: 3 in, 3 out]
  n162 = call "PECT_GateConverse.vi"("Gate 2"="Gate 2", "Gate 1"="Gate 1", "Freq_Sampling_SizeX_SizeY"=w32) -> ("Length T/2"=w33:i32, "Length"=w34:i32, "Start 2"=w35:i32, "Start 1"=w36:i32)  [unwired: 4 in, 1 out]
  n163 = Initialize Array(0.0 ("element"), w1) -> (w55:dbl[])
  n164 = Obtain Queue(name (unnamed)="data Extraction", element data type=0.0) -> (queue out=w52:refnum<queue>)  [unwired: 3 in, 2 out]
  n165 = Obtain Queue(max queue size (-1, unlimited)=10000, name (unnamed)="data DAQ", element data type=dbl[] [] ("data")) -> (queue out=w54:refnum<queue>)  [unwired: 2 in, 2 out]
  n166 = Obtain Queue(max queue size (-1, unlimited)=2 ("최대 큐 크기(-1,제한없음)"), name (unnamed)="2D data", element data type=dbl[][] [] ("initialized array")) -> (queue out=w29:refnum<queue>)  [unwired: 2 in, 2 out]
  n167 = case shown="\"                    Test mode                   \"" "Tab Control 2" {
    tunnel: w45 -> [w461 w702 w729]
    tunnel: [w460 w702 w728] -> w61
    tunnel: [w459 w701 w727] -> w60
    tunnel: w55 -> [w456 _ w726]
    tunnel: w26 -> [w458 w701 w725]
    tunnel: w33 -> [w457 _ w724]
    tunnel: w54 -> [w455 _ _]
    tunnel: w52 -> [w435 _ _]
    tunnel: w41 -> [w431 _ _]
    tunnel: w12 -> [w432 _ _]
    tunnel: w34 -> [w443 _ w722]
    tunnel: w36 -> [w442 _ w721]
    tunnel: w35 -> [w441 _ w720]
    tunnel: w42 -> [w440 _ _]
    tunnel: "Waveform" ("group name in (Untitled)") -> [w437 _ _]
    tunnel: w29 -> [w433 _ _]
    tunnel: w1 -> [_ _ w717]
    frame "                          Scan mode                      ", Default {
      # "Column"
      # "Row"
      n168 = Initialize Array(0.0 ("element"), w431, w432) -> (w448:dbl[][])
      n169 = local read "3D Surface ("() -> (w444:refnum<k7>)
      n170 = Matrix Size(0:w448) -> (1:w449:i32, 2:w450:i32)
      n171 = Decrement(x=w449) -> (x-1=w453:i32)
      n172 = Decrement(x=w450) -> (x-1=w452:i32)
      n173 = call "Surface_AxesScale.vi"("Y-axis Max"=w452, "X-axis max"=w453, "3D Surface"=w444, "Auto Scale"=FALSE) -> ()  [unwired: 8 in]
      n174 = while {
        shift-right: [w507] -> _
        shift-left: 0 -> [w509]
        shift-right: [w506] -> _
        shift-left: 0 -> [w508]
        tunnel: w435 -> [w505]
        shift-right: [w497] -> w429
        shift-left: w448 -> [w504]
        shift-right: [w500] -> _
        shift-left: TRUE ("Output Direction") -> [w501]
        tunnel: w433 -> [w499]
        tunnel: [w498] -> w434
        stop <- w502 stop-if-true
        n175 = local read "Scan"() -> (w496:bool)
        n176 = local read "Completed"() -> (w495:bool)
        n177 = Compound Arithmetic op=AND(invert w496, invert w495) -> (w494:bool)
        n178 = case shown="True" w494 {
          tunnel: w509 -> [w526 w572]
          tunnel: w508 -> [w525 w571]
          tunnel: [w524 w572] -> w507
          tunnel: [w518 w571] -> w506
          tunnel: w505 -> [w523 w564]
          tunnel: w504 -> [w522 w568]
          tunnel: [w515 w551] -> w497
          tunnel: [w521 _] -> w493
          tunnel: w501 -> [w520 w570]
          tunnel: [w519 w570] -> w500
          tunnel: w499 -> [w516 w553]
          tunnel: [w514 w564] -> w498
          frame False {
            n179 = Dequeue Element(queue=w523, timeout in ms (-1)=5000) -> (queue out=w514:refnum<queue>, element=w517:dbl)  [unwired: 1 in, 2 out]
            n180 = call "EletoMatr_1channel.vi"("Input Array X"=w522, "Input data"=w517, "In Row"=w526, "In Column"=w525, "Input Direction"=w520) -> ("Completed"=w521:bool, "Out Array X"=w515:dbl[][], "Out Row"=w524:i32, "Output Direction"=w519:bool, "Out Column"=w518:i32)  [unwired: 6 in]
            n181 = Lossy Enqueue Element(queue=w516, element=w515) -> ()  [unwired: 1 in, 4 out]
          }
          frame True {
            n182 = local read "Gate 1"() -> (w567:dbl)
            n183 = local read "Gate 2"() -> (w566:dbl)
            n184 = Wait Until Next ms Multiple(millisecond multiple=u32 100 ("ms 배수")) -> ()  [unwired: 1 out]
            n185 = local read "Offset"() -> (w558:bool)
            n186 = call "TDMS_Open.vi"("Offset"=w558, "Gate 2"=w566, "Gate 1"=w567, "Input 2D"=w568, "Open"="Open tdms") -> ("Output 2D"=w531:dbl[][])  [unwired: 5 in, 1 out]
            n187 = case shown="True" "Open tdms" {
              tunnel: w531 -> [_ w573]
              frame False {
              }
              frame True {
                n188 = global write "Global_data.vi" "global 2d graph"(w573) -> ()
              }
            }
            n189 = call "RepairLine.vi"("Repair Line Col"="Repair Line Col", "Repair Line Row"="Repair Line Row", "Line Col"="Line Col", "Line Row"="Line Row", "Array In"=w531) -> ("Array Repaired"=w545:dbl[][])  [unwired: 6 in]
            n190 = call "CSV Open.vi"("2D Array In"=w545, "Open"="Open csv") -> ("2D Array Out"=w552:dbl[][])  [unwired: 9 in]
            n191 = call "Backdata.vi"("Backindex"="Backindex", "Array in"=w552, "Backdata"="Backdata") -> ("Array out"=w534:dbl[][])
            n192 = call "TrimXY.vi"("X-max"="Y-max", "X-min"="Y-min", "Y-max"="X-max", "Y-min"="X-min", "Array In"=w534, "Trim data"="Trim data") -> ("Array Trim Out"=w533:dbl[][])  [unwired: 5 in]
            n193 = global read "Global_data.vi" "global 2d graph"() -> (w528:dbl[][])
            n194 = call "Inverse.vi"(10:"Inverse"=w533, 11:"Inverse"="Inverse") -> ("Array out"=w529:dbl[][])  [unwired: 9 in]
            n195 = call "Return data.vi"("Array Return"=w528, "Array Input"=w529, "Return"="Return") -> ("Array out"=w527:dbl[][])  [unwired: 8 in]
            n196 = call "Abs.vi"("Input"=w527, "Abs"="Abs") -> ("Array out"=w557:dbl[][])  [unwired: 9 in]
            n197 = call "DiffX.vi"("Array in"=w557, "DiffX"="DiffX") -> ("Array out"=w562:dbl[][])  [unwired: 1 in]
            n198 = call "DiffY.vi"("Array in"=w562, "DiffY"="DiffY") -> ("Array out"=w560:dbl[][])  [unwired: 1 in]
            n199 = call "Odd.vi"("Odd"="Odd", "Array In"=w560) -> ("Array Out"=w549:dbl[][])  [unwired: 9 in]
            n200 = call "Filter_Lowpass - 2D.vi"("Filter"="Filter", "Input 2D"=w549, "low cutoff freq: fl"="low cutoff freq: fl") -> ("Output"=w548:dbl[][])  [unwired: 6 in]
            n201 = case shown="True" TRUE {
              tunnel: w548 -> [w574 w575]
              tunnel: [w574 w575] -> w551
              tunnel: w553 -> [_ w576]
              frame False {
              }
              frame True {
                n202 = local read "3D Surface ("() -> (w580:refnum<k7>)
                n203 = Matrix Size(0:w575) -> (1:w581:i32, 2:w578:i32)
                n204 = Decrement(x=w581) -> (x-1=w579:i32)
                n205 = Decrement(x=w578) -> (x-1=w577:i32)
                n206 = call "Surface_AxesScale.vi"("Y-axis Max"=w577, "X-axis max"=w579, "3D Surface"=w580, "Auto Scale"=FALSE) -> ()  [unwired: 8 in]
                n207 = Lossy Enqueue Element(queue=w576, element=w575) -> ()  [unwired: 1 in, 4 out]
              }
            }
          }
        }
        "Output" <- w497
        n208 = case shown="True" w493 {
          selector: w493 -> [w510 w511]
          tunnel: [w510 w511] -> w492
          frame False {
          }
          frame True {
            n209 = Wait (ms)(milliseconds to wait=u32 200) -> ()  [unwired: 1 out]
          }
        }
        "Completed" <- w492
        n210 = local read "Exit"() -> (w503:bool)
        n211 = Compound Arithmetic op=OR(w492, w503) -> (w502:bool)
        "No. Y" <- w508
        "No. X" <- w509
      }
      n212 = while {
        tunnel: w461 -> [w591]
        tunnel: [w590] -> w460
        tunnel: [w589] -> w459
        tunnel: w458 -> [w588]
        tunnel: w455 -> [w587]
        stop <- w583 stop-if-true
        n213 = case shown="True" "Scan" {
          tunnel: w591 -> [w593 w598]
          tunnel: [w593 w597] -> w590
          tunnel: [w592 w596] -> w589
          tunnel: w588 -> [w592 w595]
          tunnel: w587 -> [_ w594]
          frame False {
          }
          frame True {
            n214 = while {
              tunnel: w598 -> [w611]
              tunnel: [w614] -> w597
              tunnel: [w613] -> w596
              tunnel: w595 -> [w610]
              tunnel: w594 -> [w612]
              stop <- w603 stop-if-true
              n215 = First Call?() -> (First Call?: T/F=w607:bool)
              n216 = case shown="True" w607 {
                tunnel: w611 -> [w615 w621]
                tunnel: w610 -> [w616 w620]
                tunnel: [w615 w619] -> w609
                tunnel: [w616 w618] -> w608
                frame False {
                }
                frame True {
                  n217 = local read "Motor Pulses"() -> (→"Init pulses":i32)
                  n218 = call <vilib>:"DAQmx Start Task.vi"("task/channels in"=w621, "error in"=w620) -> ("task out"=w619:refnum<k21>, "error out"=w618:errorcluster)  [unwired: 12 in]
                }
              }
              n219 = call-poly <vilib>:"DAQmx Read.vi"("task/channels in"=w609, "error in"=w608) -> ("task out"=w614:refnum<k21>, "data"=w601:waveform(dbl)[], "error out"=w613:errorcluster)  [unwired: 11 in]
              n220 = Index Array(array=w601, index=0 ("index (row)")) -> (element=w600:waveform(dbl))
              n221 = Unbundle By Name(w600) -> ("Y"=w599:dbl[])
              n222 = Enqueue Element(queue=w612, element=w599) -> ()  [unwired: 2 in, 3 out]
              n223 = Unbundle By Name(w613) -> ("status"=w604:bool)
              n224 = local read "Completed"() -> (w606:bool)
              n225 = local read "Exit"() -> (w605:bool)
              n226 = Compound Arithmetic op=OR(w604, w606, w605) -> (w603:bool)
            }
          }
        }
        n227 = local read "Completed"() -> (w584:bool)
        n228 = local read "Exit"() -> (w585:bool)
        n229 = Compound Arithmetic op=OR(w584, w585) -> (w583:bool)
      }
      n230 = while {
        shift-right: [w636] -> _
        shift-left: w456 -> [w640]
        tunnel: w456 -> [w639]
        tunnel: w457 -> [w638]
        tunnel: w455 -> [w637]
        tunnel: w435 -> [w635]
        shift-right: [w632] -> _
        shift-left: 0 -> [w633]
        tunnel: w443 -> [w631]
        tunnel: w442 -> [w630]
        tunnel: w441 -> [w629]
        tunnel: w440 -> [w628]
        tunnel: [w627] -> w439
        tunnel: [w626] -> w438
        tunnel: w437 -> [w625]
        stop <- w622 stop-if-true
        n231 = local read "Scan"() -> (w634:bool)
        n232 = case shown="True" w634 {
          tunnel: w640 -> [w644 w655]
          tunnel: w639 -> [_ w661]
          tunnel: w638 -> [_ w660]
          tunnel: w637 -> [_ w659]
          tunnel: [w644 w658] -> w636
          tunnel: w635 -> [_ w657]
          tunnel: w633 -> [w643 w653]
          tunnel: [w643 w652] -> w632
          tunnel: w631 -> [_ w651]
          tunnel: w630 -> [_ w650]
          tunnel: w629 -> [_ w649]
          tunnel: w628 -> [w641 w648]
          tunnel: [w641 w647] -> w627
          tunnel: [_ w646] -> w626
          tunnel: w625 -> [_ w645]
          frame False {
            n233 = Wait Until Next ms Multiple(millisecond multiple=u32 100 ("ms 배수")) -> ()  [unwired: 1 out]
          }
          frame True {
            n234 = local read "Pulser Cycles"() -> (w654:i32)
            n235 = Increment(x=w653) -> (x+1=w652:i32)
            n236 = Dequeue Element(queue=w659) -> (element=w656:dbl[])  [unwired: 2 in, 3 out]
            n237 = Quotient & Remainder(x=w652, y=w654) -> (x-y*floor(x/y)=w662:i32)  [unwired: 1 out]
            n238 = Add(x=w656, y=w655) -> (x+y=w664:dbl[])
            n239 = Equal To 0?(x=w662) -> (x = 0?=w663:bool)
            n240 = case shown="True" w663 {
              tunnel: w654 -> [_ w689]
              tunnel: w664 -> [w666 w687]
              tunnel: [w666 w690] -> w658
              tunnel: w661 -> [_ w690]
              tunnel: w660 -> [_ w683]
              tunnel: w657 -> [_ w688]
              tunnel: w651 -> [_ w684]
              tunnel: w650 -> [_ w686]
              tunnel: w649 -> [_ w685]
              tunnel: w648 -> [w665 w681]
              tunnel: [w665 w679] -> w647
              tunnel: [_ w678] -> w646
              tunnel: w645 -> [_ w680]
              frame False {
                n241 = disable-structure shown="Enabled" {
                  frame Disabled {
                    n242 = Wait Until Next ms Multiple(millisecond multiple=u32 100 ("ms 배수")) -> ()  [unwired: 1 out]
                  }
                  frame Enabled {
                  }
                }
              }
              frame True {
                n243 = Divide(x=w687, y=w689) -> (x/y=w672:dbl[])
                n244 = local read "Start idx"() -> (w671:i32)
                n245 = local read "End idx"() -> (w676:i32)
                n246 = local read "Offset"() -> (w682:bool)
                n247 = Subtract(x=w676, y=w671) -> (x-y=w673:i32)
                n248 = call "PECT_Feature extraction.vi"("Length T/2"=w683, "Offset"=w682, "Length"=w684, "Start 2"=w685, "Start 1"=w686, "Pulse signal in"=w672) -> ("Feature extraction out"=w668:dbl)  [unwired: 5 in]
                n249 = Array Subset(array=w672, index=w671, length=w673) -> (w670:dbl[])
                n250 = Absolute Value(x=w670) -> (abs(x)=w669:dbl[])
                n251 = Array Size(array=w670) -> (size(s)=w674:i32)
                n252 = Add Array Elements(numeric array=w669) -> (sum=w675:dbl)
                n253 = local read "Get data"() -> (w677:bool)
                n254 = Divide(x=w675, y=w674) -> ()  [unwired: 1 out]
                n255 = case shown="True" w677 {
                  tunnel: w688 -> [_ w699]
                  tunnel: w668 -> [_ w698]
                  tunnel: w681 -> [w691 w697]
                  tunnel: w680 -> [_ w696]
                  tunnel: w672 -> [_ w692]
                  tunnel: [w691 w695] -> w679
                  tunnel: [_ w694] -> w678
                  frame False {
                  }
                  frame True {
                    n256 = TDMS Write(0:w697, 5:w696, 9:w692) -> (4:w695:refnum<k34>, 15:w694:errorcluster)  [unwired: 3 in, 2 out]
                    n257 = Enqueue Element(queue=w699, element=w698) -> ()  [unwired: 2 in, 3 out]
                    n258 = local write "Get data"(FALSE ("Acquire")) -> ()
                  }
                }
              }
            }
          }
        }
        n259 = local read "Completed"() -> (w624:bool)
        n260 = local read "Exit"() -> (w623:bool)
        n261 = Compound Arithmetic op=OR(w624, w623) -> (w622:bool)
        "No.data" <- w633
      }
      n262 = while {
        tunnel: w433 -> [w489]
        tunnel: w432 -> [_]
        tunnel: w431 -> [_]
        tunnel: [w486] -> w430
        stop <- w487 stop-if-true
        n263 = local read "Output"() -> (w477:dbl[][])
        n264 = local read "No. Y"() -> (w484:i32)
        n265 = call "CursorPosition.vi"("Cursor No."=1.0, "Cursor"="Cursor", "3D Surface Analysis"="3D Surface (") -> ("Cursor Y"=w479:dbl)  [unwired: 6 in, 2 out]
        n266 = Dequeue Element(queue=w489, timeout in ms (-1)=3000) -> (queue out=w486:refnum<queue>)  [unwired: 1 in, 3 out]
        n267 = Add(x=w484, y=w479) -> (x+y=w483:dbl)
        n268 = Index Array(array=w477, index (col)=w483) -> (element=→"Feature extraction scan":dbl[])  [unwired: 1 in]
        n269 = call <vilib>:"3D Surface.vi"("z matrix"=w477, "3D graph"="3D Surface (") -> ()  [unwired: 8 in, 2 out]
        n270 = local read "Completed"() -> (w485:bool)
        n271 = local read "Exit"() -> (w488:bool)
        n272 = Compound Arithmetic op=OR(w485, w488) -> (w487:bool)
        n273 = Wait Until Next ms Multiple(millisecond multiple=u32 100 ("ms 배수")) -> ()  [unwired: 1 out]
      }
      n274 = Release Queue(queue=w430) -> ()  [unwired: 2 in, 3 out]
      n275 = while {
        stop <- w462 stop-if-true
        n276 = event shown="[0] \"Plot style\", \"ViewMode\": Value Change" {
          selector: _ -> [_ _ _]
          dyn-events: _ -> [_ _ _]
          timeout: _ -> [_ _ _]
          tunnel: [_ w466 _] -> w462
          event "Plot style", "ViewMode": Value Change {
            n277 = event-data() -> ()  [unwired: 1 in, 2 out]
            n278 = local read "3D Surface ("() -> (w465:refnum<k7>)
            n279 = property class="CWGraph3D"(reference=w465, "ViewMode"="ViewMode") -> ()  [unwired: 1 in, 2 out]
            n280 = call <vilib>:"Basic Properties.vi"("3D graph"=w465, "plot style"="Plot style") -> ()  [unwired: 12 in, 2 out]
          }
          event "Exit": Value Change {
            n281 = event-data() -> ()  [unwired: 1 in, 1 out]
            n282 = local read "Exit"() -> (w466:bool)
          }
          event "Max", "Min", "ColorMapAutoScale": Value Change {
            n283 = event-data() -> ()  [unwired: 1 in, 5 out]
            n284 = local read "3D Surface ("() -> (w467:refnum<k7>)
            n285 = call "Surface_ColorScale.vi"("ColorMapAutoScale"="ColorMapAutoScale", "Min"="Min", "Max"="Max", "3D Surface_"=w467) -> ("Min 2"=w471:dbl, "Max 2"=w470:dbl)  [unwired: 1 in, 2 out]
            n286 = local write "Max"(w470) -> ()
            n287 = local write "Min"(w471) -> ()
          }
        }
      }
      n288 = TDMS Close(8:w438, 11:w439) -> (0:w436:errorcluster)  [unwired: 1 out]
      n289 = call <vilib>:"Simple Error Handler.vi"("error in (no error)"=w436) -> ()  [unwired: 2 in, 7 out]
      n290 = Release Queue(queue=w434) -> ()  [unwired: 2 in, 3 out]
      n291 = while {
        tunnel: w429 -> [w475]
        stop <- w474 stop-if-true
        n292 = call "CSV Save.vi"("Array"=w475, "Save Button"="Save Scan mode") -> ()  [unwired: 9 in, 1 out]
        n293 = Wait Until Next ms Multiple(millisecond multiple=u32 100 ("ms 배수")) -> ()  [unwired: 1 out]
        n294 = local read "Exit"() -> (w474:bool)
      }
    }
    frame "Lift-Off" {
      n295 = while {
        shift-right: [w711] -> _
        shift-left: "2D Array In" -> [w712]
        stop <- w716 stop-if-true
        n296 = call "CSV Open.vi"("2D Array In"=w712, "Open"="Open") -> ("2D Array Out"=w711:dbl[][])  [unwired: 9 in]
        n297 = Delete From Array(array=w711, index (col)=0 ("disabled index (col)")) -> (array with subset deleted=w713:dbl[][])  [unwired: 2 in, 1 out]
        n298 = Subtract(x=w713, y=w711) -> (x-y=w709:dbl[][])
        n299 = Transpose 2D Array(2D array=w709) -> (transposed array=w706:dbl[][])
        n300 = call "Filter_Lowpass - 2D.vi"("Filter"="Filter lf", "Input 2D"=w706, "low cutoff freq: fl"="Low cutoff freq: fl") -> ("Output"=w708:dbl[][])  [unwired: 6 in]
        n301 = Transpose 2D Array(2D array=w708) -> (transposed array=w705:dbl[][])
        n302 = Select(t=w705, s="View Mode", f=w711) -> (s? t:f=→"Hall sensors signal lf":dbl[][])
        n303 = local read "Exit"() -> (w716:bool)
      }
    }
    frame "                    Test mode                   " {
      n304 = while {
        tunnel: w729 -> [w753]
        tunnel: w725 -> [w752]
        tunnel: [w770] -> w727
        tunnel: [w771] -> w728
        shift-right: [w766] -> _
        shift-left: w726 -> [w767]
        tunnel: w726 -> [w765]
        shift-right: [w763] -> _
        shift-left: _ -> [w762]
        tunnel: w724 -> [w761]
        shift-right: [w760] -> _
        shift-left: _ -> [w759]
        shift-right: [w757] -> _
        shift-left: 1 ("Average") -> [w756]
        tunnel: w722 -> [w749]
        tunnel: w721 -> [w748]
        tunnel: w720 -> [w747]
        shift-right: [w740] -> _
        shift-left: dbl[][] [] -> [w741]
        shift-right: [w735] -> _
        shift-left: dbl[] [] -> [w734]
        tunnel: w717 -> [w730]
        stop <- w772 stop-if-true
        n305 = First Call?() -> (First Call?: T/F=w754:bool)
        n306 = case shown="True" w754 {
          tunnel: w753 -> [w773 w778]
          tunnel: w752 -> [w774 w777]
          tunnel: [w773 w776] -> w751
          tunnel: [w774 w775] -> w750
          frame False {
          }
          frame True {
            n307 = call <vilib>:"DAQmx Start Task.vi"("task/channels in"=w778, "error in"=w777) -> ("task out"=w776:refnum<k21>, "error out"=w775:errorcluster)  [unwired: 12 in]
          }
        }
        n308 = local read "Pulser Cycles"() -> (w755:i32)
        n309 = call-poly <vilib>:"DAQmx Read.vi"("task/channels in"=w751, "number of samples per channel"=w730, "error in"=w750) -> ("task out"=w771:refnum<k21>, "data"=w732:waveform(dbl)[], "error out"=w770:errorcluster)  [unwired: 10 in]
        n310 = Quotient & Remainder(x=w756, y=w755) -> (x-y*floor(x/y)=w768:i32)  [unwired: 1 out]
        n311 = Equal To 0?(x=w768) -> (x = 0?=w746:bool)
        n312 = Index Array(array=w732, index=2 ("index (row)")) -> (element=→"Hall sensors signal 2":waveform(dbl))
        n313 = Index Array(array=w732, index #1=0 ("index (row)"), index #2=1 ("index")) -> (element #1=w744:waveform(dbl), element #2=w742:waveform(dbl))
        n314 = Unbundle By Name(w744) -> ("Y"=w736:dbl[])
        n315 = Add Array Elements(numeric array=w736) -> (sum=w738:dbl)
        n316 = Array Size(array=w736) -> (size(s)=w737:i32)
        n317 = Divide(x=w738, y=w737) -> (x/y=w739:dbl)
        n318 = Subtract(x=w736, y=w739) -> ()  [unwired: 1 out]
        n319 = Add(x=w736, y=w767) -> (x+y=w764:dbl[])
        n320 = case shown="True" w746 {
          tunnel: w755 -> [_ w823]
          tunnel: w744 -> [_ w819]
          tunnel: w764 -> [w785 w828]
          tunnel: [w785 w827] -> w766
          tunnel: w765 -> [_ w827]
          tunnel: [w784 w801] -> w763
          tunnel: w762 -> [w784 w826]
          tunnel: w761 -> [_ w814]
          tunnel: [w783 w824] -> w760
          tunnel: w759 -> [w783 w825]
          tunnel: [w781 1 ("Average")] -> w757
          tunnel: w756 -> [w782 _]
          tunnel: w749 -> [_ w815]
          tunnel: w748 -> [_ w817]
          tunnel: w747 -> [_ w816]
          tunnel: w742 -> [_ _]
          tunnel: [w780 w808] -> w740
          tunnel: w741 -> [w780 w807]
          tunnel: [w779 w794] -> w735
          tunnel: w734 -> [w779 w793]
          frame False {
            n321 = Increment(x=w782) -> (x+1=w781:i32)
          }
          frame True {
            n322 = Divide(x=w828, y=w823) -> (x/y=w792:dbl[])
            n323 = call "PECT_Feature extraction.vi"("Length T/2"=w814, "Offset"="Offset", "Length"=w815, "Start 2"=w816, "Start 1"=w817, "Pulse signal in"=w792) -> ()  [unwired: 5 in, 1 out]
            n324 = case shown="True" "Backdata" {
              tunnel: w792 -> [w829 w832]
              tunnel: [w829 w830] -> w794
              tunnel: w793 -> [_ w830]
              tunnel: [w829 w831] -> w789
              frame False {
              }
              frame True {
                n325 = Subtract(x=w832, y=w830) -> (x-y=w831:dbl[])
              }
            }
            n326 = call "Filter_Lowpass.vi"("Filter"="Filter 2", "Pulse signal in"=w789, "low cutoff freq: fl"="low cutoff freq: fl 2") -> ("Signal out"=w788:dbl[])  [unwired: 6 in]
            n327 = Bundle By Name(cluster=w819, "Y"=w788) -> (w800:waveform(dbl))
            n328 = call-poly <vilib>:"FFT Power Spectrum and PSD.vi"("time signal"=w800) -> ("Power Spectrum / PSD"=w799:cluster{"f0":dbl, "df":dbl, "magnitude":dbl[]})  [unwired: 7 in, 3 out]
            n329 = case shown="True" "2 Plots" {
              tunnel: [w840 w846] -> w786
              tunnel: w826 -> [_ w845]
              tunnel: [w837 w845] -> w801
              tunnel: w800 -> [w837 w841]
              tunnel: w799 -> [w838 w843]
              tunnel: [w839 w844] -> w820
              tunnel: w825 -> [_ w842]
              tunnel: [w838 w842] -> w824
              frame False {
                n330 = Build Array(w838, w838) -> (w839:cluster{"f0":dbl, "df":dbl, "magnitude":dbl[]}[])
                n331 = Build Array(w837, w837) -> (w840:waveform(dbl)[])
              }
              frame True {
                n332 = Build Array(w842, w843) -> (w844:cluster{"f0":dbl, "df":dbl, "magnitude":dbl[]}[])
                n333 = Build Array(w845, w841) -> (w846:waveform(dbl)[])
              }
            }
            "Power spectral density" <- w820
            "Hall sensors signal" <- w786
            n334 = case shown="True" "Add LF" {
              tunnel: w788 -> [_ w836]
              tunnel: [w833 w834] -> w808
              tunnel: w807 -> [w833 w835]
              frame False {
              }
              frame True {
                n335 = Build Array (concatenate)(w835, w836) -> (w834:dbl[][])
              }
            }
            "Array" <- w808
            n336 = call "CSV Save.vi"("Array"=w808, "Save Button"="Save LF") -> ("Save Status"=→"Save Status":bool)  [unwired: 9 in]
            n337 = Subtract(x="End idx", y="Start idx") -> (x-y=w802:i32)
            n338 = Array Subset(array=w788, index="Start idx", length=w802) -> (w797:dbl[])
            n339 = Square(x=w797) -> (x^2=w796:dbl[])
            n340 = Delete From Array(array=w808, index (col)=0 ("disabled index (col)")) -> (array with subset deleted=w809:dbl[][])  [unwired: 2 in, 1 out]
            n341 = Array Size(array=w797) -> (size(s)=w805:i32)
            n342 = Add Array Elements(numeric array=w796) -> (sum=w806:dbl)
            n343 = Divide(x=w806, y=w805) -> (x/y=→"Feature Extraction":dbl)
            n344 = Subtract(x=w809, y=w808) -> (x-y=→"dy":dbl[][])
          }
        }
        n345 = local read "Exit"() -> (w758:bool)
        n346 = Unbundle By Name(w770) -> ("status"=w769:bool)
        n347 = Or(x=w769, y=w758) -> (x .or. y?=w772:bool)
      }
    }
  }
  n348 = disable-structure shown="Disabled" {
    disable-tunnel: w19 -> [w850 _]
    disable-tunnel: w18 -> [w849 _]
    disable-tunnel: w17 -> [w848 _]
    disable-tunnel: w16 -> [w847 _]
    frame Disabled {
      # "Update. Pos X"
      # "Mov. dis Y"
      # "Old. Pos Y"
      # "Mov. dis X"
      # "Old. Pos X"
      n349 = while {
        shift-right: [w879] -> _
        shift-left: T1."No Scan" -> [w884]
        shift-right: [w875] -> _
        shift-left: 0.0 ("Current  Position (mm)") -> [w883]
        shift-right: [w876] -> _
        shift-left: 0.0 ("Current  Position (mm)") -> [w882]
        shift-right: [w874] -> _
        shift-left: 0.0 ("Current  Position (mm)") -> [w881]
        shift-right: [w873] -> _
        shift-left: 0.0 ("Current  Position (mm)") -> [w880]
        tunnel: w848 -> [w878]
        tunnel: w847 -> [w865]
        tunnel: w850 -> [w877]
        tunnel: w849 -> [w864]
        tunnel: [w872] -> _
        tunnel: [w870] -> w856
        tunnel: [w871] -> _
        tunnel: [w869] -> w857
        shift-right: [w862] -> _
        shift-left: 0.0 ("Current  Position (mm)") -> [w861]
        stop <- w866 stop-if-true
        n350 = case shown="\"Wait X\"" w884 {
          selector: w884 -> [w903 _ _ _ _]
          tunnel: w883 -> [w896 w963 w985 w1049 w1089]
          tunnel: w882 -> [w897 w962 w991 w1048 w1088]
          tunnel: w881 -> [_ w961 w1008 w1029 w1072]
          tunnel: w880 -> [_ w960 w1009 w1047 w1070]
          tunnel: [w902 T1."Wait X" w987 w1040 w1074] -> w879
          tunnel: w878 -> [w901 w955 w1004 w1038 w1083]
          tunnel: w865 -> [w900 w956 w1005 w1039 w1084]
          tunnel: w877 -> [w899 w957 w997 w1034 w1086]
          tunnel: w864 -> [w898 w958 w998 w1035 w1085]
          tunnel: [w889 w962 w991 w1048 w1088] -> w876
          tunnel: [w888 w963 w988 w1049 w1089] -> w875
          tunnel: [w891 w961 w1008 w1029 w1087] -> w874
          tunnel: [w890 w960 w1009 w1047 w1070] -> w873
          tunnel: [w895 w949 w1002 w1037 w1081] -> w872
          tunnel: [w894 w948 w1000 w1036 w1079] -> w870
          tunnel: [w893 w947 w1006 w1032 w1077] -> w871
          tunnel: [w892 w946 w1007 w1033 w1075] -> w869
          tunnel: w865 -> [_ _ _ _ _]
          tunnel: [w887 w945 w978 w1027 w1066] -> w862
          tunnel: w861 -> [w886 w945 w984 w1027 w1066]
          frame "No Scan", Default {
            n351 = local read "Scan"() -> (w885:bool)
            n352 = case shown="True" w885 {
              tunnel: w903 -> [w911 _]
              tunnel: [w911 w922] -> w902
              tunnel: w901 -> [w908 w920]
              tunnel: w900 -> [w909 w919]
              tunnel: w899 -> [w906 w918]
              tunnel: w898 -> [w907 w917]
              tunnel: w897 -> [w905 _]
              tunnel: w896 -> [w910 _]
              tunnel: [w910 w916] -> w888
              tunnel: [w909 w926] -> w895
              tunnel: [w908 w925] -> w894
              tunnel: [w907 w924] -> w893
              tunnel: [w906 w923] -> w892
              tunnel: [w905 w921] -> w891
              tunnel: [w904 w916] -> w887
              tunnel: w886 -> [w904 _]
              frame False {
              }
              frame True {
                n353 = flat-sequence {
                  tunnel: w917 -> [w927]
                  tunnel: w918 -> [w928]
                  tunnel: w919 -> [w929]
                  tunnel: w920 -> [w930]
                  tunnel: [w930] -> w915
                  tunnel: [w929] -> w914
                  tunnel: [w928] -> w913
                  tunnel: [w927] -> w912
                  tunnel: [w944] -> w926
                  tunnel: [w943] -> w925
                  tunnel: [w942] -> w924
                  tunnel: [w941] -> w923
                  tunnel: [T1."Move X"] -> w922
                  tunnel: [w939] -> w921
                  tunnel: [w932] -> w916
                  tunnel: w915 -> [w938]
                  tunnel: w914 -> [w937]
                  tunnel: w913 -> [w936]
                  tunnel: w912 -> [w935]
                  frame #0 {
                  }
                  frame #1 {
                    n354 = local write "Direction (+)"("+" ("Direction (+)")) -> ()
                    n355 = local write "Numeric"(0.0 ("Numeric")) -> ()
                    n356 = local read "Travel per Pulse (mm)"() -> (w934:dbl)
                    n357 = call "Autonics_GetPos.vi"("error in (no error)"=w938, "Travel per Pulse (mm)"=w934, "VISA resource name"=w937) -> ("error out"=w943:errorcluster, "Current  Position (mm)"=w932:dbl, "VISA resource name out"=w944:refnum<visa-resource-name>)  [unwired: 6 in]
                    "Start Pos Y" <- w932
                    n358 = call "Autonics_GetPos.vi"("error in (no error)"=w936, "Travel per Pulse (mm)"=w934, "VISA resource name"=w935) -> ("error out"=w941:errorcluster, "Current  Position (mm)"=w939:dbl, "VISA resource name out"=w942:refnum<visa-resource-name>)  [unwired: 6 in]
                    "Start Pos X" <- w939
                    n359 = local write "Cur. Pos X"(w932) -> ()
                    n360 = local write "Cur. Pos Y"(w939) -> ()
                  }
                }
              }
            }
            n361 = local read "X - length"() -> (w889:dbl)
            n362 = local read "Step Y"() -> (w890:dbl)
          }
          frame "Move X" {
            n363 = local read "Travel per Pulse (mm)"() -> (w950:dbl)
            n364 = local read "X - length"() -> (w951:dbl)
            n365 = call "Autonics_Move.vi"("Direction (+)"="Direction (+)", "error in (no error)"=w955, "Travel per Pulse (mm)"=w950, "Move Distance (mm)"=w951, "VISA resource name"=w956) -> ("error out"=w953:errorcluster, "VISA resource name out"=w954:refnum<visa-resource-name>)  [unwired: 5 in]
            n366 = flat-sequence {
              tunnel: [w968] -> w949
              tunnel: w954 -> [w968]
              tunnel: [w967] -> w948
              tunnel: w953 -> [w967]
              tunnel: [w965] -> w947
              tunnel: w958 -> [w965]
              tunnel: [w964] -> w946
              tunnel: w957 -> [w964]
              frame #0 {
                n367 = Wait (ms)(milliseconds to wait=u32 100) -> ()  [unwired: 1 out]
              }
            }
          }
          frame "Wait X" {
            n368 = local read "Travel per Pulse (mm)"() -> (w995:dbl)
            n369 = call "Autonics_GetPos.vi"("error in (no error)"=w997, "Travel per Pulse (mm)"=w995, "VISA resource name"=w998) -> ("error out"=w996:errorcluster, "Current  Position (mm)"=w994:dbl, "VISA resource name out"=w999:refnum<visa-resource-name>)  [unwired: 6 in]
            n370 = call "Autonics_GetPos.vi"("error in (no error)"=w1004, "Travel per Pulse (mm)"=w995, "VISA resource name"=w1005) -> ("error out"=w1001:errorcluster, "Current  Position (mm)"=w976:dbl, "VISA resource name out"=w1003:refnum<visa-resource-name>)  [unwired: 6 in]
            n371 = local read "Direction (+)"() -> (w971:string)
            n372 = local write "Cur. Pos Y"(w994) -> ()
            n373 = Equal?(x=w971, y="-") -> (x = y?=w969:bool)
            n374 = local read "Step X"() -> (w981:dbl)
            n375 = local write "Cur. Pos X"(w976) -> ()
            n376 = Subtract(x=w976, y=w984) -> (x-y=w983:dbl)
            n377 = Absolute Value(x=w991) -> (abs(x)=w993:dbl)
            n378 = Absolute Value(x=w983) -> (abs(x)=w982:dbl)
            n379 = Subtract(x=w976, y=w985) -> (x-y=w992:dbl)
            n380 = Greater Or Equal?(x=w982, y=w981) -> (x >= y?=w977:bool)
            n381 = Quotient & Remainder(x=w976, y=w981) -> (floor(x/y)=w973:dbl)  [unwired: 1 out]
            n382 = Absolute Value(x=w992) -> (abs(x)=w986:dbl)
            n383 = Subtract(x=w986, y=w993) -> (x-y=w989:dbl)
            n384 = case shown="True" w977 {
              selector: w977 -> [_ w1010]
              frame False {
              }
              frame True {
                n385 = local read "Numeric"() -> (w1012:dbl)
                n386 = Increment(x=w1012) -> (x+1=→"Numeric":dbl)
                "Acquire" <- w1010
              }
            }
            n387 = Increment(x=w973) -> (x+1=w974:dbl)
            n388 = call "Convert Double Precision.vi"("Input"=w989) -> ("Output"=w990:dbl)  [unwired: 10 in]
            n389 = Select(t=w974, s=w969, f=w973) -> (s? t:f=w972:dbl)
            n390 = Multiply(x=w972, y=w981) -> (x*y=w980:dbl)
            n391 = Select(t=w980, s=w977, f=w984) -> (s? t:f=w979:dbl)
            n392 = Greater Or Equal To 0?(x=w990) -> (x >= 0?=w975:bool)
            n393 = Select(t=w976, s=w975, f=w979) -> (s? t:f=w978:dbl)
            n394 = case shown="True" w975 {
              tunnel: [w1015 w1026] -> w1007
              tunnel: w996 -> [w1015 w1026]
              tunnel: [w1016 w1025] -> w1006
              tunnel: w999 -> [w1016 w1025]
              tunnel: [w1018 w1024] -> w1002
              tunnel: w1003 -> [w1018 w1024]
              tunnel: [w1017 w1023] -> w1000
              tunnel: w1001 -> [w1017 w1023]
              tunnel: [w1014 w1022] -> w988
              tunnel: w985 -> [w1014 _]
              tunnel: [T1."Wait X" T1."Move Y"] -> w987
              frame False {
              }
              frame True {
                n395 = local read "Cur. Pos X"() -> (w1022:dbl)
                n396 = local write "Numeric"(0.0 ("Numeric")) -> ()
                n397 = Wait (ms)(milliseconds to wait=u32 1000) -> ()  [unwired: 1 out]
              }
            }
            "Current  Position (mm)" <- w984
          }
          frame "Move Y" {
            n398 = local read "Step Y"() -> (w1043:dbl)
            n399 = local read "Y - length"() -> (w1028:dbl)
            n400 = local read "Start Pos Y"() -> (w1030:dbl)
            n401 = Subtract(x=w1028, y=w1043) -> ()  [unwired: 1 out]
            n402 = Subtract(x=w1030, y=w1029) -> (x-y=w1046:dbl)
            n403 = Absolute Value(x=w1028) -> (abs(x)=w1044:dbl)
            n404 = Absolute Value(x=w1046) -> (abs(x)=w1045:dbl)
            n405 = Subtract(x=w1045, y=w1044) -> (x-y=w1042:dbl)
            n406 = call "Convert Double Precision.vi"("Input"=w1042) -> ("Output"=w1041:dbl)  [unwired: 10 in]
            n407 = Greater Or Equal To 0?(x=w1041) -> (x >= 0?=w1031:bool)
            n408 = case shown="True" w1031 {
              tunnel: [T1."Wait Y" T1."No Scan"] -> w1040
              tunnel: w1039 -> [w1057 w1063]
              tunnel: [w1058 w1062] -> w1036
              tunnel: w1038 -> [w1058 w1062]
              tunnel: [w1057 w1063] -> w1037
              tunnel: w1035 -> [w1051 w1061]
              tunnel: w1034 -> [w1055 w1060]
              tunnel: [w1056 w1060] -> w1033
              tunnel: [w1050 w1061] -> w1032
              frame False {
                n409 = local read "Step Y"() -> (w1054:dbl)
                n410 = local read "Travel per Pulse (mm)"() -> (w1052:dbl)
                n411 = call "Autonics_Move.vi"("Direction (+)"="+" ("Direction (+) 2"), "error in (no error)"=w1055, "Travel per Pulse (mm)"=w1052, "Move Distance (mm)"=w1054, "VISA resource name"=w1051) -> ("error out"=w1056:errorcluster, "VISA resource name out"=w1050:refnum<visa-resource-name>)  [unwired: 5 in]
              }
              frame True {
                n412 = local write "Scan"(FALSE) -> ()
              }
            }
          }
          frame "Wait Y" {
            n413 = local read "Travel per Pulse (mm)"() -> (w1067:dbl)
            n414 = call "Autonics_GetPos.vi"("error in (no error)"=w1086, "Travel per Pulse (mm)"=w1067, "VISA resource name"=w1085) -> ("error out"=w1076:errorcluster, "Current  Position (mm)"=w1071:dbl, "VISA resource name out"=w1078:refnum<visa-resource-name>)  [unwired: 6 in]
            n415 = call "Autonics_GetPos.vi"("error in (no error)"=w1083, "Travel per Pulse (mm)"=w1067, "VISA resource name"=w1084) -> ("error out"=w1080:errorcluster, "Current  Position (mm)"=w1073:dbl, "VISA resource name out"=w1082:refnum<visa-resource-name>)  [unwired: 6 in]
            n416 = Subtract(x=w1071, y=w1072) -> (x-y=w1091:dbl)
            n417 = Absolute Value(x=w1070) -> (abs(x)=w1093:dbl)
            n418 = Absolute Value(x=w1091) -> (abs(x)=w1092:dbl)
            n419 = Subtract(x=w1092, y=w1093) -> (x-y=w1090:dbl)
            n420 = local write "Cur. Pos X"(w1073) -> ()
            n421 = local write "Cur. Pos Y"(w1071) -> ()
            n422 = call "Convert Double Precision.vi"("Input"=w1090) -> ("Output"=w1069:dbl)  [unwired: 10 in]
            n423 = Greater Or Equal To 0?(x=w1069) -> (x >= 0?=w1068:bool)
            n424 = case shown="True" w1068 {
              tunnel: w1072 -> [w1099 _]
              tunnel: [w1099 w1112] -> w1087
              tunnel: w1082 -> [w1098 w1110]
              tunnel: [w1098 w1110] -> w1081
              tunnel: [w1097 w1109] -> w1079
              tunnel: w1080 -> [w1097 w1109]
              tunnel: [w1096 w1108] -> w1077
              tunnel: w1078 -> [w1096 w1108]
              tunnel: [w1095 w1107] -> w1075
              tunnel: w1076 -> [w1095 w1107]
              tunnel: [T1."Wait Y" T1."Move X"] -> w1074
              frame False {
              }
              frame True {
                n425 = local read "Direction (+)"() -> (w1106:string)
                n426 = local read "Cur. Pos Y"() -> (w1112:dbl)
                n427 = Equal?(x=w1106, y="+") -> (x = y?=w1104:bool)
                n428 = Select(t="-", s=w1104, f="+") -> (s? t:f=w1103:string)
                n429 = local write "Direction (+)"(w1103) -> ()
                n430 = Wait (ms)(milliseconds to wait=u32 1000) -> ()  [unwired: 1 out]
              }
            }
          }
        }
        n431 = Wait Until Next ms Multiple(millisecond multiple=u32 100 ("milliseconds to wait")) -> ()  [unwired: 1 out]
        n432 = local read "Completed"() -> (w860:bool)
        n433 = local read "Exit"() -> (w859:bool)
        n434 = Unbundle By Name(w869) -> ("status"=w867:bool)
        n435 = Unbundle By Name(w870) -> ("status"=w868:bool)
        n436 = Compound Arithmetic op=OR(w860, w859, w868, w867) -> (w866:bool)
        "Enum" <- w884
      }
      n437 = call <vilib>:"Simple Error Handler.vi"("error in (no error)"=w856) -> ()  [unwired: 4 in, 5 out]
      n438 = call <vilib>:"Simple Error Handler.vi"("error in (no error)"=w857) -> ()  [unwired: 4 in, 5 out]
    }
    frame Enabled {
    }
  }
  n439 = call <vilib>:"DAQmx Clear Task.vi"("task in"=w61, "error in"=w60) -> ("error out"=w67:errorcluster)  [unwired: 13 in]
  n440 = call <vilib>:"Simple Error Handler.vi"("error in (no error)"=w67) -> ()  [unwired: 4 in, 5 out]
  n441 = call <vilib>:"Simple Error Handler.vi"() -> ()  [unwired: 5 in, 5 out]
